vi "32路模拟量输入.vi"() -> ()   [LabVIEW 2010]
uses:
  全局量/全局_配置.vi
panel:
  in  "同步_1":i32
  in  "数组_反馈值":dbl[][](array[numeric])
  in  "第几个数据":i32
  in  "第几组数据":i32
  out "数组_AD幅值":sgl[](array[numeric])
  out "数组_DSP幅值":sgl[](array[numeric])
  in  "数组_设定值":dbl[][](array[numeric])
  in  "数组_选择":bool[](array[boolean])
  out "light_32":bool
  out "light_31":bool
  out "light_30":bool
  out "light_29":bool
  out "light_28":bool
  out "light_27":bool
  out "light_26":bool
  out "light_25":bool
  out "light_24":bool
  out "light_23":bool
  out "light_22":bool
  out "light_21":bool
  out "light_20":bool
  out "light_19":bool
  out "light_18":bool
  out "light_17":bool
  out "Analog_back":string[][](table) caption="表格"
  in  "A_32":bool
  in  "A_31":bool
  in  "A_30":bool
  in  "A_29":bool
  in  "A_28":bool
  in  "A_27":bool
  in  "A_26":bool
  in  "A_25":bool
  in  "A_24":bool
  in  "A_23":bool
  in  "A_22":bool
  in  "A_21":bool
  in  "A_20":bool
  in  "A_19":bool
  in  "A_18":bool
  in  "A_17":bool
  out "合格？":bool[][](array[boolean])
  out "测试结论":string
  out "light_16":bool
  out "light_15":bool
  out "light_14":bool
  out "light_13":bool
  out "light_12":bool
  out "light_11":bool
  out "light_10":bool
  out "light_9":bool
  out "light_8":bool
  out "light_7":bool
  out "light_6":bool
  out "light_5":bool
  out "light_4":bool
  out "light_3":bool
  out "light_2":bool
  out "light_1":bool
  out "退出？":bool
  in  "btn_反选":bool
  in  "btn_全选":bool
  in  "A_16":bool
  in  "A_15":bool
  in  "A_14":bool
  in  "A_13":bool
  in  "A_12":bool
  in  "A_11":bool
  in  "A_10":bool
  in  "A_9":bool
  in  "A_8":bool
  in  "A_7":bool
  in  "A_6":bool
  in  "A_5":bool
  in  "A_4":bool
  in  "A_3":bool
  in  "A_2":bool
  in  "A_1":bool
  in  "btn_取消":bool
  in  "btn_开始测试":bool
  in  "Analog_IN":string[][](table) caption="表格"
  out "Analog_WC":string[][](table) caption="表格"
  # "模拟量选择及输入值（V）"
  # "模拟量反馈值（V）"
  # "模拟量误差值（%）"
  # "测试结论："
  # "从0开始"
  # "从1开始,第0列没有使用"
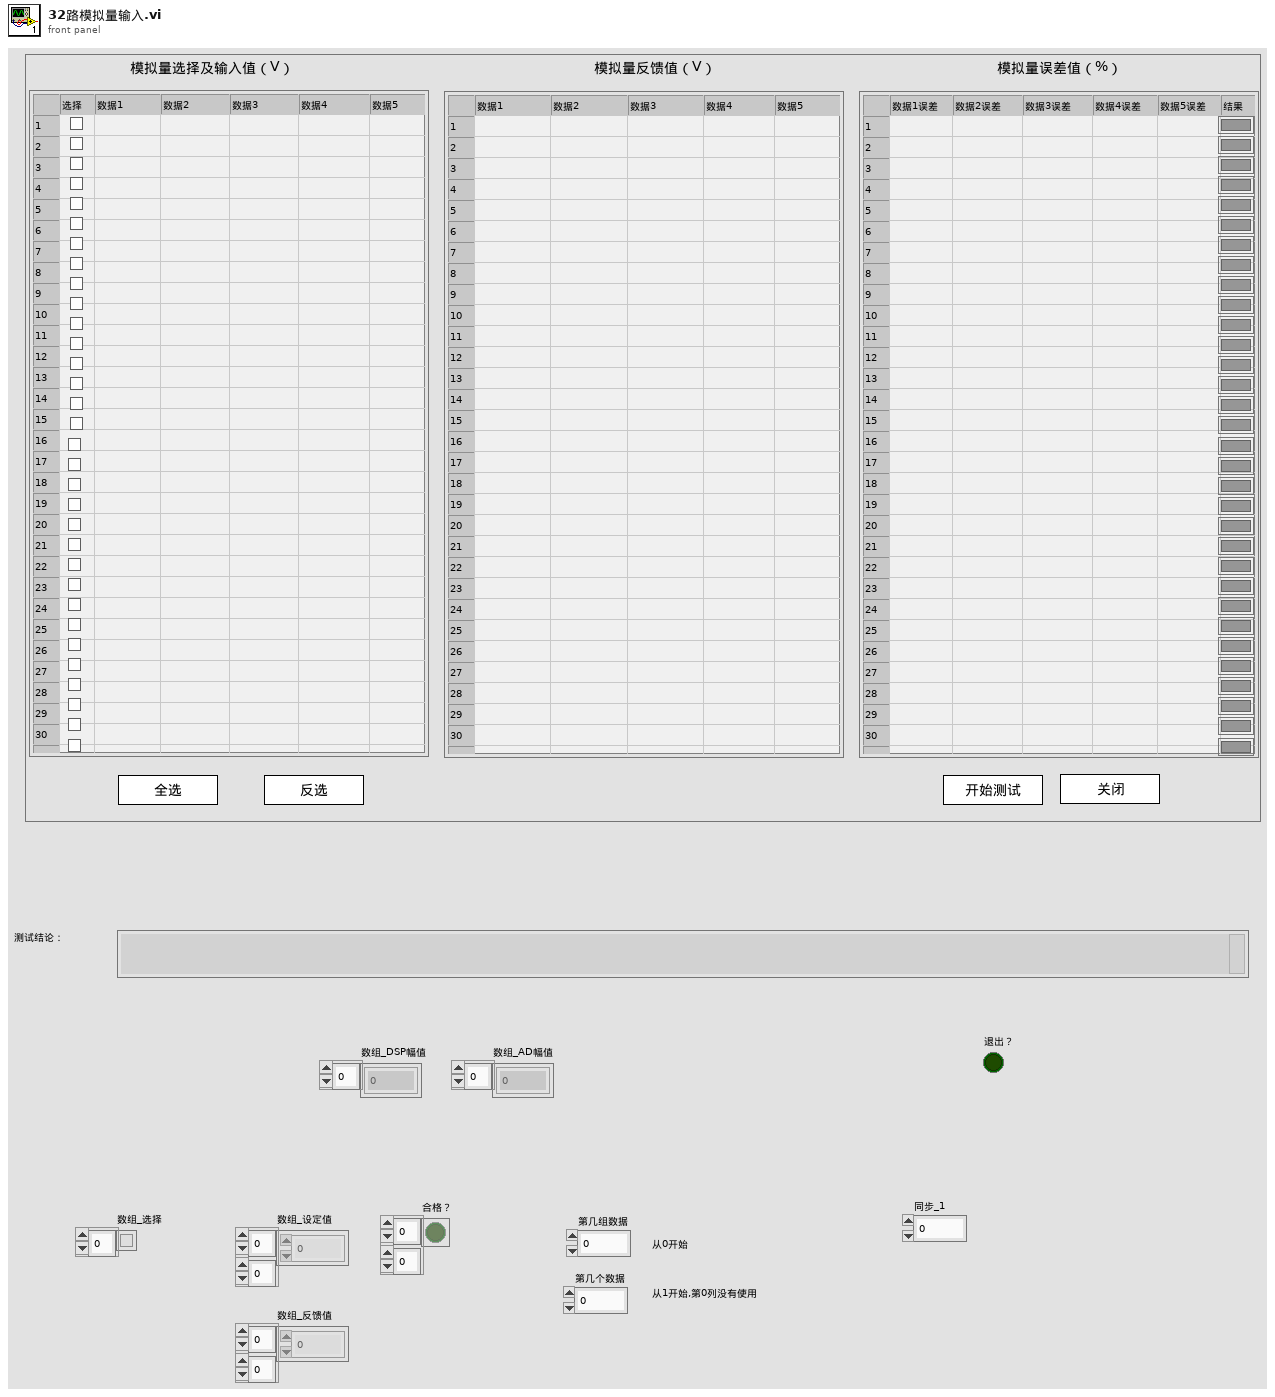
[diagram p1: front panel]
types:
  T1 = enum8{"Enabled", "Disabled", "Disabled and Grayed Out"}
  T2 = cluster{"数字量输入信号路数":u32, "数字量输出信号路数":u32, "DSP模拟量输入信号路数":u32, "DSP模拟量输入信号幅值":u32, "AD模拟量输入信号路数":u32, "AD模拟量输入信号幅值":u32, "RS232端口":i32, "RS232通信路数":u32, "RS232波特率":u32, "RS485端口":u32, "RS485通信路数":u32, "RS485波特率":u32, "CAN通信路数":i32, "CAN波特率":u32, "以太网选择?":bool, "控制板IP":string, "以太网端口":u32}
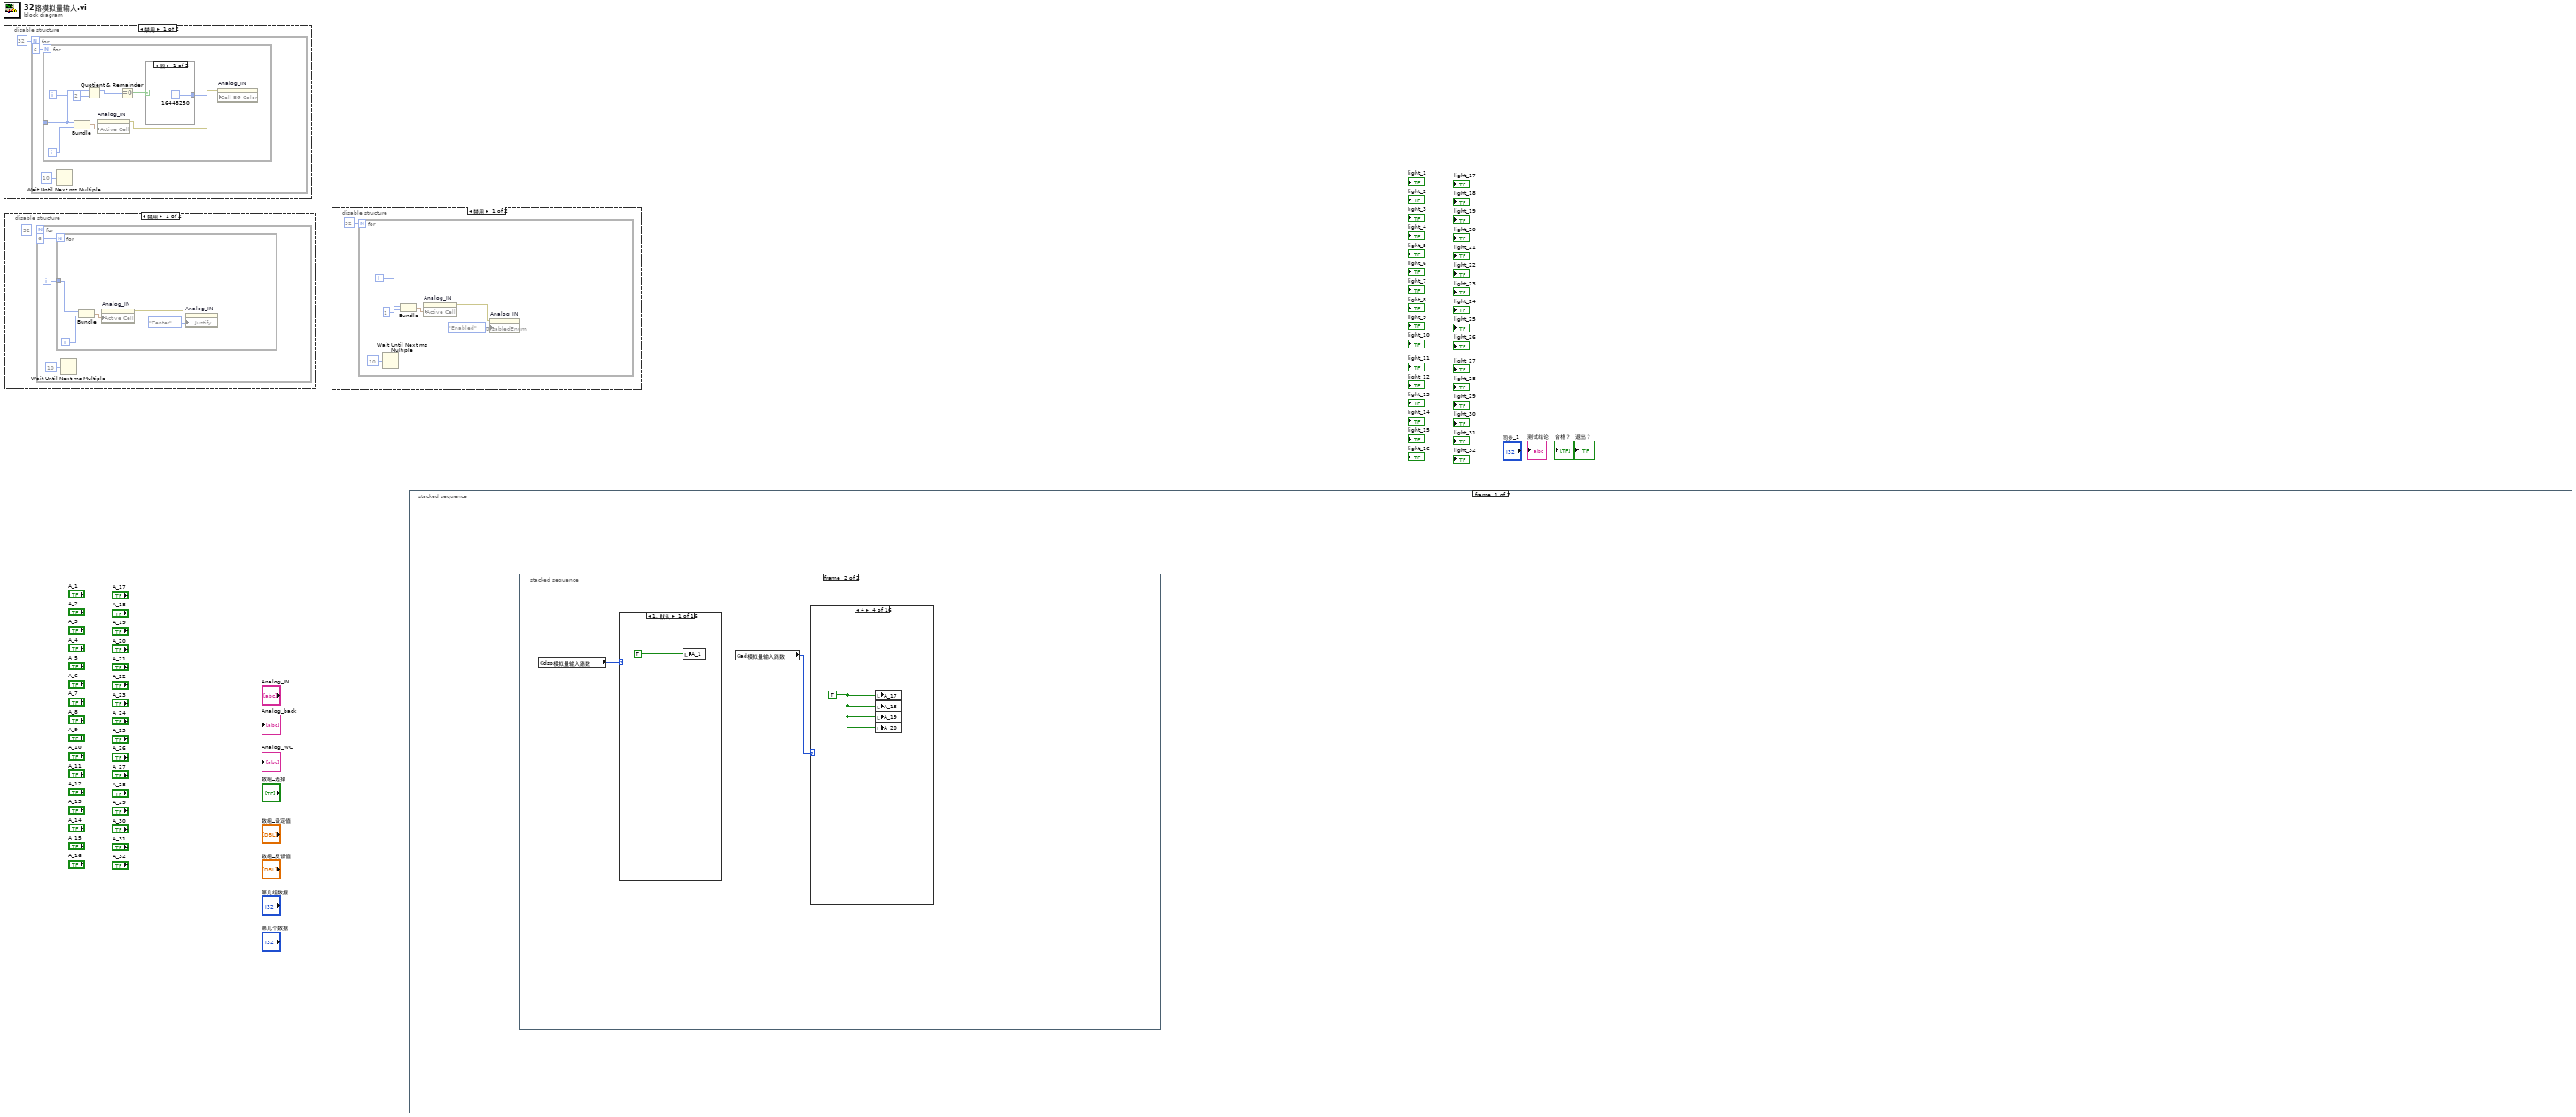
[diagram p0: block diagram]
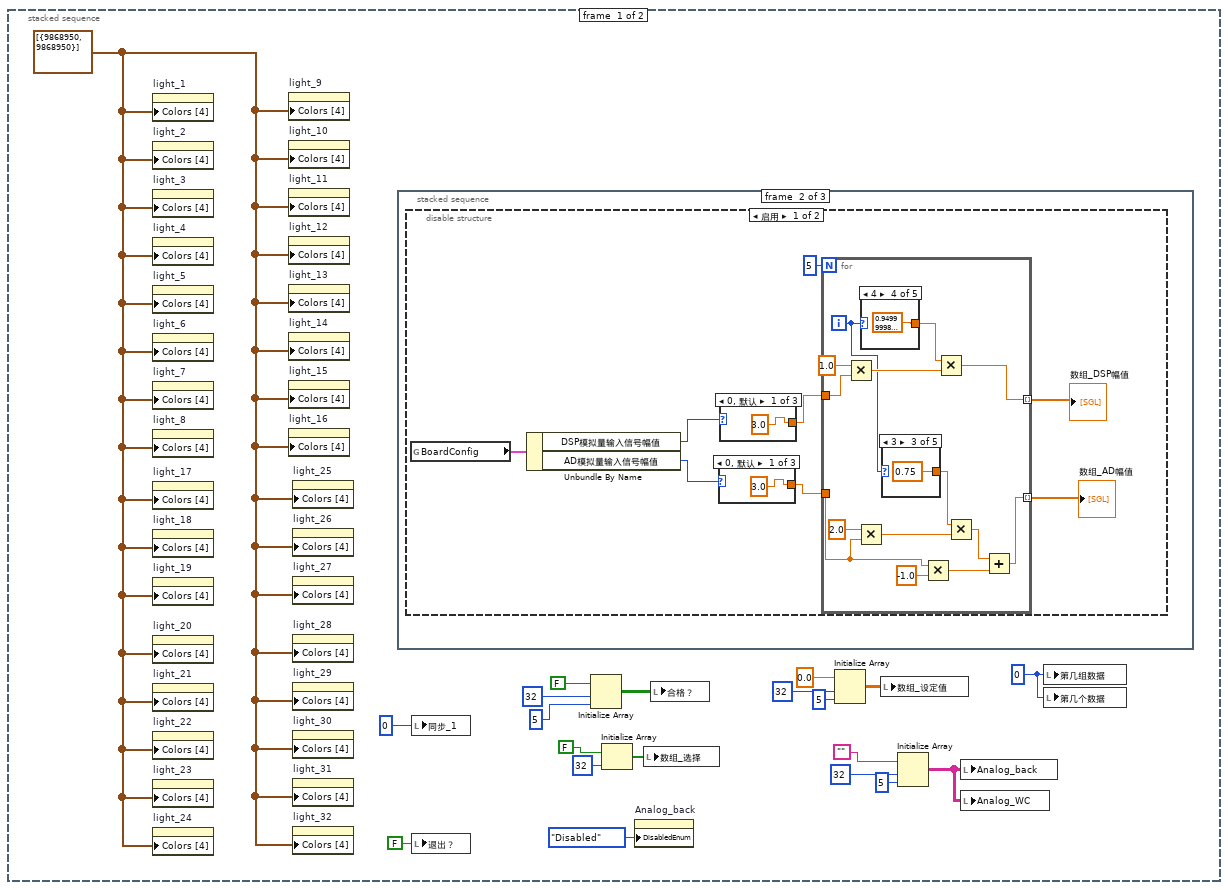
[diagram p2: hidden frame]
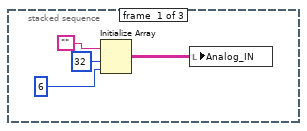
[diagram p3: hidden frame]
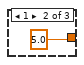
[diagram p4: hidden frame]
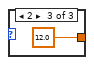
[diagram p5: hidden frame]
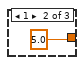
[diagram p6: hidden frame]
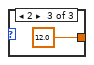
[diagram p7: hidden frame]
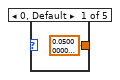
[diagram p8: hidden frame]
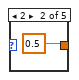
[diagram p9: hidden frame]
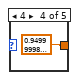
[diagram p10: hidden frame]
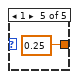
[diagram p11: hidden frame]
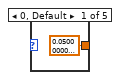
[diagram p12: hidden frame]
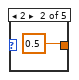
[diagram p13: hidden frame]
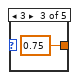
[diagram p14: hidden frame]
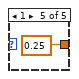
[diagram p15: hidden frame]
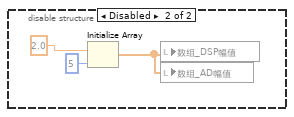
[diagram p16: hidden frame]
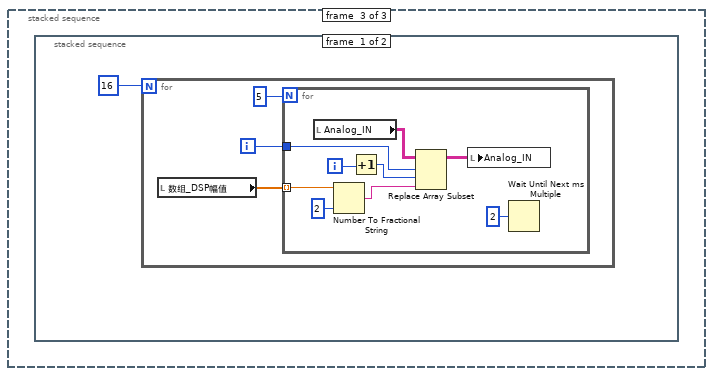
[diagram p17: hidden frame]
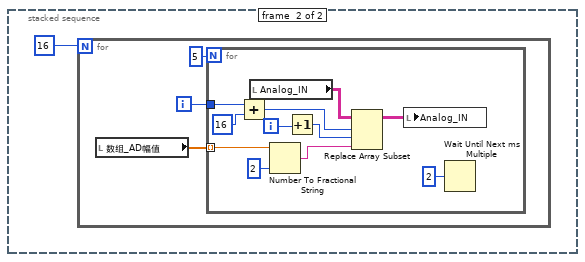
[diagram p18: hidden frame]
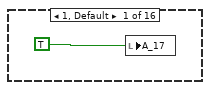
[diagram p19: hidden frame]
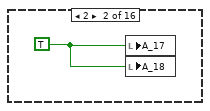
[diagram p20: hidden frame]
diagram:
  n1 = disable-structure shown="禁用" {
    frame Disabled {
      n2 = for {
        N: 32 -> [_]
        i -> [w3]
        n3 = for {
          N: 6 -> [_]
          tunnel: w3 -> [w11]
          i -> [w5]
          n4 = Bundle(w11, w5) -> (w8:cluster{i32, i32})  [unwired: 1 in]
          n5 = Quotient & Remainder(x=w11, y=2) -> (x-y*floor(x/y)=w9:i32)  [unwired: 1 out]
          n6 = property on="Analog_IN" class="Tbl (严格)"("Active Cell"=w8) -> (error out=w7:errorcluster)  [unwired: 2 in, 1 out]
          n7 = Equal To 0?(x=w9) -> (x = 0?=w12:bool)
          n8 = case shown="假" w12 {
            tunnel: [u32 16448250 u32 15723488] -> w6
            frame False {
            }
            frame True {
            }
          }
          n9 = property on="Analog_IN" class="Tbl (严格)"(error in=w7, "Cell BG Color"=w6) -> ()  [unwired: 1 in, 2 out]
        }
        n10 = Wait Until Next ms Multiple(millisecond multiple=u32 10 ("毫秒倍数")) -> ()  [unwired: 1 out]
      }
    }
    frame Enabled {
    }
  }
  n11 = disable-structure shown="禁用" {
    frame Disabled {
      n12 = for {
        N: 32 -> [_]
        i -> [w16]
        n13 = for {
          N: 6 -> [_]
          tunnel: w16 -> [w19]
          i -> [w20]
          n14 = Bundle(w19, w20) -> (w23:cluster{i32, i32})  [unwired: 1 in]
          n15 = property on="Analog_IN" class="Tbl (严格)"("Active Cell"=w23) -> (error out=w21:errorcluster)  [unwired: 2 in, 1 out]
          n16 = property on="Analog_IN" class="Tbl (严格)"(error in=w21, "Justify"=enum16{"Left", "Center", "Right"}."Center" ("活动单元格:单元格对齐")) -> ()  [unwired: 1 in, 2 out]
        }
        n17 = Wait Until Next ms Multiple(millisecond multiple=u32 10 ("毫秒倍数")) -> ()  [unwired: 1 out]
      }
    }
    frame Enabled {
    }
  }
  n18 = disable-structure shown="禁用" {
    frame Disabled {
      n19 = for {
        N: 32 -> [_]
        i -> [w29]
        n20 = Wait Until Next ms Multiple(millisecond multiple=u32 10 ("毫秒倍数")) -> ()  [unwired: 1 out]
        n21 = Bundle(w29, 1) -> (w28:cluster{i32, i32})  [unwired: 1 in]
        n22 = property on="Analog_IN" class="Tbl (严格)"("Active Cell"=w28) -> (error out=w25:errorcluster)  [unwired: 2 in, 1 out]
        n23 = property on="Analog_IN" class="Tbl (严格)"(error in=w25, "DisabledEnum"=T1."Enabled" ("禁用")) -> ()  [unwired: 1 in, 2 out]
      }
    }
    frame Enabled {
    }
  }
  n24 = stacked-sequence {
    frame #0 {
      n25 = stacked-sequence {
        frame #0 {
          w31 = 0 ("第几组数据")
          w46 = cluster{u32, u32}[] [{9868950, 9868950}]
          n26 = property on="light_1" class="Bool (严格)"("Colors [4]"=w46) -> ()  [unwired: 2 in, 2 out]
          n27 = property on="light_2" class="Bool (严格)"("Colors [4]"=w46) -> ()  [unwired: 2 in, 2 out]
          n28 = property on="light_3" class="Bool (严格)"("Colors [4]"=w46) -> ()  [unwired: 2 in, 2 out]
          n29 = property on="light_4" class="Bool (严格)"("Colors [4]"=w46) -> ()  [unwired: 2 in, 2 out]
          n30 = property on="light_5" class="Bool (严格)"("Colors [4]"=w46) -> ()  [unwired: 2 in, 2 out]
          n31 = property on="light_6" class="Bool (严格)"("Colors [4]"=w46) -> ()  [unwired: 2 in, 2 out]
          n32 = property on="light_7" class="Bool (严格)"("Colors [4]"=w46) -> ()  [unwired: 2 in, 2 out]
          n33 = property on="light_8" class="Bool (严格)"("Colors [4]"=w46) -> ()  [unwired: 2 in, 2 out]
          n34 = property on="light_17" class="Bool (严格)"("Colors [4]"=w46) -> ()  [unwired: 2 in, 2 out]
          n35 = property on="light_18" class="Bool (严格)"("Colors [4]"=w46) -> ()  [unwired: 2 in, 2 out]
          n36 = property on="light_19" class="Bool (严格)"("Colors [4]"=w46) -> ()  [unwired: 2 in, 2 out]
          n37 = property on="light_20" class="Bool (严格)"("Colors [4]"=w46) -> ()  [unwired: 2 in, 2 out]
          n38 = property on="light_21" class="Bool (严格)"("Colors [4]"=w46) -> ()  [unwired: 2 in, 2 out]
          n39 = property on="light_22" class="Bool (严格)"("Colors [4]"=w46) -> ()  [unwired: 2 in, 2 out]
          n40 = property on="light_23" class="Bool (严格)"("Colors [4]"=w46) -> ()  [unwired: 2 in, 2 out]
          n41 = property on="light_24" class="Bool (严格)"("Colors [4]"=w46) -> ()  [unwired: 2 in, 2 out]
          n42 = property on="light_9" class="Bool (严格)"("Colors [4]"=w46) -> ()  [unwired: 2 in, 2 out]
          n43 = property on="light_10" class="Bool (严格)"("Colors [4]"=w46) -> ()  [unwired: 2 in, 2 out]
          n44 = property on="light_11" class="Bool (严格)"("Colors [4]"=w46) -> ()  [unwired: 2 in, 2 out]
          n45 = property on="light_12" class="Bool (严格)"("Colors [4]"=w46) -> ()  [unwired: 2 in, 2 out]
          n46 = property on="light_13" class="Bool (严格)"("Colors [4]"=w46) -> ()  [unwired: 2 in, 2 out]
          n47 = property on="light_14" class="Bool (严格)"("Colors [4]"=w46) -> ()  [unwired: 2 in, 2 out]
          n48 = property on="light_15" class="Bool (严格)"("Colors [4]"=w46) -> ()  [unwired: 2 in, 2 out]
          n49 = property on="light_16" class="Bool (严格)"("Colors [4]"=w46) -> ()  [unwired: 2 in, 2 out]
          n50 = property on="light_25" class="Bool (严格)"("Colors [4]"=w46) -> ()  [unwired: 2 in, 2 out]
          n51 = property on="light_26" class="Bool (严格)"("Colors [4]"=w46) -> ()  [unwired: 2 in, 2 out]
          n52 = property on="light_27" class="Bool (严格)"("Colors [4]"=w46) -> ()  [unwired: 2 in, 2 out]
          n53 = property on="light_28" class="Bool (严格)"("Colors [4]"=w46) -> ()  [unwired: 2 in, 2 out]
          n54 = property on="light_29" class="Bool (严格)"("Colors [4]"=w46) -> ()  [unwired: 2 in, 2 out]
          n55 = property on="light_30" class="Bool (严格)"("Colors [4]"=w46) -> ()  [unwired: 2 in, 2 out]
          n56 = property on="light_31" class="Bool (严格)"("Colors [4]"=w46) -> ()  [unwired: 2 in, 2 out]
          n57 = property on="light_32" class="Bool (严格)"("Colors [4]"=w46) -> ()  [unwired: 2 in, 2 out]
          n58 = stacked-sequence {
            frame #0 {
              n59 = Initialize Array("", 32 ("维数大小"), 6 ("维数大小")) -> (w51:string[][])
              n60 = local write "Analog_IN"(w51) -> ()
            }
            frame #1 {
              n61 = disable-structure shown="启用" {
                frame Enabled {
                  n62 = global read "全局_配置.vi" "BoardConfig"() -> (w59:T2)
                  n63 = Unbundle By Name(w59) -> ("DSP模拟量输入信号幅值"=w58:u32, "AD模拟量输入信号幅值"=w57:u32)
                  n64 = case shown="0, 默认" w57 {
                    tunnel: [sgl 3.0 sgl 5.0 sgl 12.0] -> w55
                    frame 0, Default {
                    }
                    frame 1 {
                    }
                    frame 2 {
                    }
                  }
                  n65 = case shown="0, 默认" w58 {
                    tunnel: [sgl 3.0 sgl 5.0 sgl 12.0] -> w56
                    frame 0, Default {
                    }
                    frame 1 {
                    }
                    frame 2 {
                    }
                  }
                  n66 = for {
                    N: 5 -> [_]
                    tunnel: w56 -> [w82]
                    tunnel: w55 -> [w74]
                    tunnel: [w69] -> w61 mode=indexing
                    tunnel: [w72] -> w60 mode=indexing
                    i -> [w71]
                    n67 = Multiply(x=sgl 1.0, y=w82) -> (x*y=w80:sgl)
                    n68 = Multiply(x=sgl 2.0, y=w74) -> (x*y=w78:sgl)
                    n69 = case shown="4" w71 {
                      tunnel: [sgl 0.05 sgl 0.5 sgl 0.75 sgl 0.95 sgl 0.25] -> w73
                      frame 0, Default {
                      }
                      frame 2 {
                      }
                      frame 3 {
                      }
                      frame 4 {
                      }
                      frame 1 {
                      }
                    }
                    n70 = case shown="3" w71 {
                      tunnel: [sgl 0.05 sgl 0.5 sgl 0.75 sgl 0.95 sgl 0.25] -> w70
                      frame 0, Default {
                      }
                      frame 2 {
                      }
                      frame 3 {
                      }
                      frame 4 {
                      }
                      frame 1 {
                      }
                    }
                    n71 = Multiply(x=w74, y=sgl -1.0) -> (x*y=w76:sgl)
                    n72 = Multiply(x=w73, y=w80) -> (x*y=w69:sgl)
                    n73 = Multiply(x=w70, y=w78) -> (x*y=w79:sgl)
                    n74 = Add(x=w79, y=w76) -> (x+y=w72:sgl)
                  }
                  "数组_DSP幅值" <- w61
                  "数组_AD幅值" <- w60
                }
                frame Disabled {
                  n75 = Initialize Array(sgl 2.0, 5 ("维数大小")) -> (w95:sgl[])
                  n76 = local write "数组_DSP幅值"(w95) -> ()
                  n77 = local write "数组_AD幅值"(w95) -> ()
                }
              }
            }
            frame #2 {
              n78 = stacked-sequence {
                frame #0 {
                  n79 = for {
                    N: 16 -> [_]
                    i -> [w97]
                    n80 = local read "数组_DSP幅值"() -> (w98:sgl[])
                    n81 = for {
                      N: 5 -> [_]
                      tunnel: w98 -> [w105] mode=indexing
                      tunnel: w97 -> [w104]
                      i -> [w102]
                      n82 = local read "Analog_IN"() -> (w108:string[][])
                      n83 = Number To Fractional String(number=w105, precision (6)=i16 2 ("精度(6)")) -> (F-format string=w103:string)  [unwired: 2 in]
                      n84 = Increment(x=w102) -> (x+1=w101:i32)
                      n85 = Replace Array Subset(array=w108, new element=w103, index (row)=w104, index (col)=w101) -> (w107:string[][])
                      n86 = local write "Analog_IN"(w107) -> ()
                      n87 = Wait Until Next ms Multiple(millisecond multiple=u32 2 ("毫秒倍数")) -> ()  [unwired: 1 out]
                    }
                  }
                }
                frame #1 {
                  n88 = for {
                    N: 16 -> [_]
                    i -> [w111]
                    n89 = local read "数组_AD幅值"() -> (w110:sgl[])
                    n90 = for {
                      N: 5 -> [_]
                      tunnel: w110 -> [w120] mode=indexing
                      tunnel: w111 -> [w115]
                      i -> [w118]
                      n91 = Add(x=w115, y=16) -> (x+y=w113:i32)
                      n92 = local read "Analog_IN"() -> (w123:string[][])
                      n93 = Number To Fractional String(number=w120, precision (6)=i16 2 ("精度(6)")) -> (F-format string=w119:string)  [unwired: 2 in]
                      n94 = Increment(x=w118) -> (x+1=w117:i32)
                      n95 = Replace Array Subset(array=w123, new element=w119, index (row)=w113, index (col)=w117) -> (w122:string[][])
                      n96 = local write "Analog_IN"(w122) -> ()
                      n97 = Wait Until Next ms Multiple(millisecond multiple=u32 2 ("毫秒倍数")) -> ()  [unwired: 1 out]
                    }
                  }
                }
              }
            }
          }
          n98 = local write "同步_1"(0 ("同步_2")) -> ()
          n99 = local write "退出？"(FALSE ("退出？")) -> ()
          n100 = Initialize Array(FALSE, 32 ("维数大小"), 5 ("维数大小")) -> (w47:bool[][])
          n101 = Initialize Array(FALSE, 32 ("维数大小")) -> (w35:bool[])
          n102 = property on="Analog_back" class="Tbl (严格)"("DisabledEnum"=T1."Disabled" ("禁用")) -> ()  [unwired: 2 in, 2 out]
          n103 = local write "数组_选择"(w35) -> ()
          n104 = local write "合格？"(w47) -> ()
          n105 = Initialize Array(0.0, 32 ("维数大小"), 5 ("维数大小")) -> (w38:dbl[][])
          n106 = local write "数组_设定值"(w38) -> ()
          n107 = Initialize Array("", 32 ("维数大小"), 5 ("维数大小")) -> (w42:string[][])
          n108 = local write "Analog_back"(w42) -> ()
          n109 = local write "Analog_WC"(w42) -> ()
          n110 = local write "第几组数据"(w31) -> ()
          n111 = local write "第几个数据"(w31) -> ()
        }
        frame #1 {
          n112 = global read "全局_配置.vi" "dsp模拟量输入路数"() -> (w125:u32)
          n113 = case shown="1, 默认" w125 {
            frame 1, Default {
              n114 = local write "A_1"(TRUE ("单选_AD_1")) -> ()
            }
            frame 2 {
              w143 = TRUE ("单选_AD_1")
              n115 = local write "A_1"(w143) -> ()
              n116 = local write "A_2"(w143) -> ()
            }
            frame 3 {
              w144 = TRUE ("单选_AD_1")
              n117 = local write "A_1"(w144) -> ()
              n118 = local write "A_2"(w144) -> ()
              n119 = local write "A_3"(w144) -> ()
            }
            frame 4 {
              w145 = TRUE ("单选_AD_1")
              n120 = local write "A_1"(w145) -> ()
              n121 = local write "A_2"(w145) -> ()
              n122 = local write "A_3"(w145) -> ()
              n123 = local write "A_4"(w145) -> ()
            }
            frame 5 {
              w146 = TRUE ("单选_AD_1")
              n124 = local write "A_1"(w146) -> ()
              n125 = local write "A_2"(w146) -> ()
              n126 = local write "A_3"(w146) -> ()
              n127 = local write "A_4"(w146) -> ()
              n128 = local write "A_5"(w146) -> ()
            }
            frame 6 {
              w147 = TRUE ("单选_AD_1")
              n129 = local write "A_1"(w147) -> ()
              n130 = local write "A_2"(w147) -> ()
              n131 = local write "A_3"(w147) -> ()
              n132 = local write "A_4"(w147) -> ()
              n133 = local write "A_5"(w147) -> ()
              n134 = local write "A_6"(w147) -> ()
            }
            frame 7 {
              w148 = TRUE ("单选_AD_1")
              n135 = local write "A_1"(w148) -> ()
              n136 = local write "A_2"(w148) -> ()
              n137 = local write "A_3"(w148) -> ()
              n138 = local write "A_4"(w148) -> ()
              n139 = local write "A_5"(w148) -> ()
              n140 = local write "A_6"(w148) -> ()
              n141 = local write "A_7"(w148) -> ()
            }
            frame 8 {
              w149 = TRUE ("单选_AD_1")
              n142 = local write "A_1"(w149) -> ()
              n143 = local write "A_2"(w149) -> ()
              n144 = local write "A_3"(w149) -> ()
              n145 = local write "A_4"(w149) -> ()
              n146 = local write "A_5"(w149) -> ()
              n147 = local write "A_6"(w149) -> ()
              n148 = local write "A_7"(w149) -> ()
              n149 = local write "A_8"(w149) -> ()
            }
            frame 9 {
              w150 = TRUE ("单选_AD_1")
              n150 = local write "A_1"(w150) -> ()
              n151 = local write "A_2"(w150) -> ()
              n152 = local write "A_3"(w150) -> ()
              n153 = local write "A_4"(w150) -> ()
              n154 = local write "A_5"(w150) -> ()
              n155 = local write "A_6"(w150) -> ()
              n156 = local write "A_7"(w150) -> ()
              n157 = local write "A_8"(w150) -> ()
              n158 = local write "A_9"(w150) -> ()
            }
            frame 10 {
              w151 = TRUE ("单选_AD_1")
              n159 = local write "A_1"(w151) -> ()
              n160 = local write "A_2"(w151) -> ()
              n161 = local write "A_3"(w151) -> ()
              n162 = local write "A_4"(w151) -> ()
              n163 = local write "A_5"(w151) -> ()
              n164 = local write "A_6"(w151) -> ()
              n165 = local write "A_7"(w151) -> ()
              n166 = local write "A_8"(w151) -> ()
              n167 = local write "A_9"(w151) -> ()
              n168 = local write "A_10"(w151) -> ()
            }
            frame 11 {
              w152 = TRUE ("单选_AD_1")
              n169 = local write "A_1"(w152) -> ()
              n170 = local write "A_2"(w152) -> ()
              n171 = local write "A_3"(w152) -> ()
              n172 = local write "A_4"(w152) -> ()
              n173 = local write "A_5"(w152) -> ()
              n174 = local write "A_6"(w152) -> ()
              n175 = local write "A_7"(w152) -> ()
              n176 = local write "A_8"(w152) -> ()
              n177 = local write "A_9"(w152) -> ()
              n178 = local write "A_10"(w152) -> ()
              n179 = local write "A_11"(w152) -> ()
            }
            frame 12 {
              w153 = TRUE ("单选_AD_1")
              n180 = local write "A_1"(w153) -> ()
              n181 = local write "A_2"(w153) -> ()
              n182 = local write "A_3"(w153) -> ()
              n183 = local write "A_4"(w153) -> ()
              n184 = local write "A_5"(w153) -> ()
              n185 = local write "A_6"(w153) -> ()
              n186 = local write "A_7"(w153) -> ()
              n187 = local write "A_8"(w153) -> ()
              n188 = local write "A_9"(w153) -> ()
              n189 = local write "A_10"(w153) -> ()
              n190 = local write "A_11"(w153) -> ()
              n191 = local write "A_12"(w153) -> ()
            }
            frame 13 {
              w154 = TRUE ("单选_AD_1")
              n192 = local write "A_1"(w154) -> ()
              n193 = local write "A_2"(w154) -> ()
              n194 = local write "A_3"(w154) -> ()
              n195 = local write "A_4"(w154) -> ()
              n196 = local write "A_5"(w154) -> ()
              n197 = local write "A_6"(w154) -> ()
              n198 = local write "A_7"(w154) -> ()
              n199 = local write "A_8"(w154) -> ()
              n200 = local write "A_9"(w154) -> ()
              n201 = local write "A_10"(w154) -> ()
              n202 = local write "A_11"(w154) -> ()
              n203 = local write "A_12"(w154) -> ()
              n204 = local write "A_13"(w154) -> ()
            }
            frame 14 {
              w155 = TRUE ("单选_AD_1")
              n205 = local write "A_1"(w155) -> ()
              n206 = local write "A_2"(w155) -> ()
              n207 = local write "A_3"(w155) -> ()
              n208 = local write "A_4"(w155) -> ()
              n209 = local write "A_5"(w155) -> ()
              n210 = local write "A_6"(w155) -> ()
              n211 = local write "A_7"(w155) -> ()
              n212 = local write "A_8"(w155) -> ()
              n213 = local write "A_9"(w155) -> ()
              n214 = local write "A_10"(w155) -> ()
              n215 = local write "A_11"(w155) -> ()
              n216 = local write "A_12"(w155) -> ()
              n217 = local write "A_13"(w155) -> ()
              n218 = local write "A_14"(w155) -> ()
            }
            frame 15 {
              w156 = TRUE ("单选_AD_1")
              n219 = local write "A_1"(w156) -> ()
              n220 = local write "A_2"(w156) -> ()
              n221 = local write "A_3"(w156) -> ()
              n222 = local write "A_4"(w156) -> ()
              n223 = local write "A_5"(w156) -> ()
              n224 = local write "A_6"(w156) -> ()
              n225 = local write "A_7"(w156) -> ()
              n226 = local write "A_8"(w156) -> ()
              n227 = local write "A_9"(w156) -> ()
              n228 = local write "A_10"(w156) -> ()
              n229 = local write "A_11"(w156) -> ()
              n230 = local write "A_12"(w156) -> ()
              n231 = local write "A_13"(w156) -> ()
              n232 = local write "A_14"(w156) -> ()
              n233 = local write "A_15"(w156) -> ()
            }
            frame 16 {
              w157 = TRUE ("单选_AD_1")
              n234 = local write "A_1"(w157) -> ()
              n235 = local write "A_2"(w157) -> ()
              n236 = local write "A_3"(w157) -> ()
              n237 = local write "A_4"(w157) -> ()
              n238 = local write "A_5"(w157) -> ()
              n239 = local write "A_6"(w157) -> ()
              n240 = local write "A_7"(w157) -> ()
              n241 = local write "A_8"(w157) -> ()
              n242 = local write "A_9"(w157) -> ()
              n243 = local write "A_10"(w157) -> ()
              n244 = local write "A_11"(w157) -> ()
              n245 = local write "A_12"(w157) -> ()
              n246 = local write "A_13"(w157) -> ()
              n247 = local write "A_14"(w157) -> ()
              n248 = local write "A_15"(w157) -> ()
              n249 = local write "A_16"(w157) -> ()
            }
          }
          n250 = global read "全局_配置.vi" "ad模拟量输入路数"() -> (w124:u32)
          n251 = case shown="4" w124 {
            frame 1, Default {
              n252 = local write "A_17"(TRUE ("单选_AD_1")) -> ()
            }
            frame 2 {
              w127 = TRUE ("单选_AD_1")
              n253 = local write "A_17"(w127) -> ()
              n254 = local write "A_18"(w127) -> ()
            }
            frame 3 {
              w128 = TRUE ("单选_AD_1")
              n255 = local write "A_17"(w128) -> ()
              n256 = local write "A_18"(w128) -> ()
              n257 = local write "A_19"(w128) -> ()
            }
            frame 4 {
              w129 = TRUE ("单选_AD_1")
              n258 = local write "A_17"(w129) -> ()
              n259 = local write "A_18"(w129) -> ()
              n260 = local write "A_19"(w129) -> ()
              n261 = local write "A_20"(w129) -> ()
            }
            frame 5 {
              w130 = TRUE ("单选_AD_1")
              n262 = local write "A_17"(w130) -> ()
              n263 = local write "A_18"(w130) -> ()
              n264 = local write "A_19"(w130) -> ()
              n265 = local write "A_20"(w130) -> ()
              n266 = local write "A_21"(w130) -> ()
            }
            frame 6 {
              w131 = TRUE ("单选_AD_1")
              n267 = local write "A_17"(w131) -> ()
              n268 = local write "A_18"(w131) -> ()
              n269 = local write "A_19"(w131) -> ()
              n270 = local write "A_20"(w131) -> ()
              n271 = local write "A_21"(w131) -> ()
              n272 = local write "A_22"(w131) -> ()
            }
            frame 7 {
              w132 = TRUE ("单选_AD_1")
              n273 = local write "A_17"(w132) -> ()
              n274 = local write "A_18"(w132) -> ()
              n275 = local write "A_19"(w132) -> ()
              n276 = local write "A_20"(w132) -> ()
              n277 = local write "A_21"(w132) -> ()
              n278 = local write "A_22"(w132) -> ()
              n279 = local write "A_23"(w132) -> ()
            }
            frame 8 {
              w133 = TRUE ("单选_AD_1")
              n280 = local write "A_17"(w133) -> ()
              n281 = local write "A_18"(w133) -> ()
              n282 = local write "A_19"(w133) -> ()
              n283 = local write "A_20"(w133) -> ()
              n284 = local write "A_21"(w133) -> ()
              n285 = local write "A_22"(w133) -> ()
              n286 = local write "A_23"(w133) -> ()
              n287 = local write "A_24"(w133) -> ()
            }
            frame 9 {
              w134 = TRUE ("单选_AD_1")
              n288 = local write "A_17"(w134) -> ()
              n289 = local write "A_18"(w134) -> ()
              n290 = local write "A_19"(w134) -> ()
              n291 = local write "A_20"(w134) -> ()
              n292 = local write "A_21"(w134) -> ()
              n293 = local write "A_22"(w134) -> ()
              n294 = local write "A_23"(w134) -> ()
              n295 = local write "A_24"(w134) -> ()
              n296 = local write "A_25"(w134) -> ()
            }
            frame 10 {
              w135 = TRUE ("单选_AD_1")
              n297 = local write "A_17"(w135) -> ()
              n298 = local write "A_18"(w135) -> ()
              n299 = local write "A_19"(w135) -> ()
              n300 = local write "A_20"(w135) -> ()
              n301 = local write "A_21"(w135) -> ()
              n302 = local write "A_22"(w135) -> ()
              n303 = local write "A_23"(w135) -> ()
              n304 = local write "A_24"(w135) -> ()
              n305 = local write "A_25"(w135) -> ()
              n306 = local write "A_26"(w135) -> ()
            }
            frame 11 {
              w136 = TRUE ("单选_AD_1")
              n307 = local write "A_17"(w136) -> ()
              n308 = local write "A_18"(w136) -> ()
              n309 = local write "A_19"(w136) -> ()
              n310 = local write "A_20"(w136) -> ()
              n311 = local write "A_21"(w136) -> ()
              n312 = local write "A_22"(w136) -> ()
              n313 = local write "A_23"(w136) -> ()
              n314 = local write "A_24"(w136) -> ()
              n315 = local write "A_25"(w136) -> ()
              n316 = local write "A_26"(w136) -> ()
              n317 = local write "A_27"(w136) -> ()
            }
            frame 12 {
              w137 = TRUE ("单选_AD_1")
              n318 = local write "A_17"(w137) -> ()
              n319 = local write "A_18"(w137) -> ()
              n320 = local write "A_19"(w137) -> ()
              n321 = local write "A_20"(w137) -> ()
              n322 = local write "A_21"(w137) -> ()
              n323 = local write "A_22"(w137) -> ()
              n324 = local write "A_23"(w137) -> ()
              n325 = local write "A_24"(w137) -> ()
              n326 = local write "A_25"(w137) -> ()
              n327 = local write "A_26"(w137) -> ()
              n328 = local write "A_27"(w137) -> ()
              n329 = local write "A_28"(w137) -> ()
            }
            frame 13 {
              w138 = TRUE ("单选_AD_1")
              n330 = local write "A_17"(w138) -> ()
              n331 = local write "A_18"(w138) -> ()
              n332 = local write "A_19"(w138) -> ()
              n333 = local write "A_20"(w138) -> ()
              n334 = local write "A_21"(w138) -> ()
              n335 = local write "A_22"(w138) -> ()
              n336 = local write "A_23"(w138) -> ()
              n337 = local write "A_24"(w138) -> ()
              n338 = local write "A_25"(w138) -> ()
              n339 = local write "A_26"(w138) -> ()
              n340 = local write "A_27"(w138) -> ()
              n341 = local write "A_28"(w138) -> ()
              n342 = local write "A_29"(w138) -> ()
            }
            frame 14 {
              w139 = TRUE ("单选_AD_1")
              n343 = local write "A_17"(w139) -> ()
              n344 = local write "A_18"(w139) -> ()
              n345 = local write "A_19"(w139) -> ()
              n346 = local write "A_20"(w139) -> ()
              n347 = local write "A_21"(w139) -> ()
              n348 = local write "A_22"(w139) -> ()
              n349 = local write "A_23"(w139) -> ()
              n350 = local write "A_24"(w139) -> ()
              n351 = local write "A_25"(w139) -> ()
              n352 = local write "A_26"(w139) -> ()
              n353 = local write "A_27"(w139) -> ()
              n354 = local write "A_28"(w139) -> ()
              n355 = local write "A_29"(w139) -> ()
              n356 = local write "A_30"(w139) -> ()
            }
            frame 15 {
              w140 = TRUE ("单选_AD_1")
              n357 = local write "A_17"(w140) -> ()
              n358 = local write "A_18"(w140) -> ()
              n359 = local write "A_19"(w140) -> ()
              n360 = local write "A_20"(w140) -> ()
              n361 = local write "A_21"(w140) -> ()
              n362 = local write "A_22"(w140) -> ()
              n363 = local write "A_23"(w140) -> ()
              n364 = local write "A_24"(w140) -> ()
              n365 = local write "A_25"(w140) -> ()
              n366 = local write "A_26"(w140) -> ()
              n367 = local write "A_27"(w140) -> ()
              n368 = local write "A_28"(w140) -> ()
              n369 = local write "A_29"(w140) -> ()
              n370 = local write "A_30"(w140) -> ()
              n371 = local write "A_31"(w140) -> ()
            }
            frame 16 {
              w141 = TRUE ("单选_AD_1")
              n372 = local write "A_17"(w141) -> ()
              n373 = local write "A_18"(w141) -> ()
              n374 = local write "A_19"(w141) -> ()
              n375 = local write "A_20"(w141) -> ()
              n376 = local write "A_21"(w141) -> ()
              n377 = local write "A_22"(w141) -> ()
              n378 = local write "A_23"(w141) -> ()
              n379 = local write "A_24"(w141) -> ()
              n380 = local write "A_25"(w141) -> ()
              n381 = local write "A_26"(w141) -> ()
              n382 = local write "A_27"(w141) -> ()
              n383 = local write "A_28"(w141) -> ()
              n384 = local write "A_29"(w141) -> ()
              n385 = local write "A_30"(w141) -> ()
              n386 = local write "A_31"(w141) -> ()
              n387 = local write "A_32"(w141) -> ()
            }
          }
        }
      }
    }
    frame #1 {
      w159 = "ANumCheck" ("名称（未命名）")
      w161 = "DSPStart" ("名称（未命名）")
      w166 = "ANumCheck" ("名称（未命名）")
      w169 = "DSPStart" ("名称（未命名）")
      n388 = Obtain Notifier(name (unnamed)=w161, notification data type=w161) -> (notifier out=w160:refnum<notifier>)  [unwired: 2 in, 2 out]
      n389 = while {
        tunnel: w160 -> [w435]
        stop <- w436 stop-if-true
        n390 = event shown="[4] \"btn_全选\": 值改变" {
          selector: _ -> [_ _ _ _ _ _]
          dyn-events: _ -> [_ _ _ _ _ _]
          timeout: _ -> [_ _ _ _ _ _]
          tunnel: [_ TRUE TRUE _ _ _] -> w436
          tunnel: w435 -> [_ _ _ w439 _ _]
          event Timeout {
            n391 = event-data() -> ()  [unwired: 1 in, 2 out]
          }
          event Panel Close {
            n392 = event-data() -> ()  [unwired: 1 in, 3 out]
          }
          event "btn_取消": Value Change {
            n393 = event-data() -> ()  [unwired: 1 in, 5 out]
          }
          event "btn_开始测试": Value Change {
            n394 = event-data() -> ()  [unwired: 1 in, 5 out]
            n395 = stacked-sequence {
              tunnel: w439 -> [_ _ _ w518]
              frame #0 {
                w440 = 0 ("第几组数据")
                n396 = local read "Analog_IN"() -> (w447:string[][])
                n397 = Delete From Array(array=w447, length=1 ("长度"), index (col)=0 ("禁用的索引 (列)")) -> (array with subset deleted=w443:string[][])  [unwired: 1 in, 1 out]
                n398 = for {
                  N: 32 -> [_]
                  tunnel: w443 -> [w450] mode=indexing
                  tunnel: [w449] -> w446 mode=indexing
                  n399 = for {
                    N: 5 -> [_]
                    tunnel: w450 -> [w452] mode=indexing
                    tunnel: [w451] -> w449 mode=indexing
                    n400 = Fract/Exp String To Number(string=w452) -> (number=w451:dbl)  [unwired: 3 in, 1 out]
                  }
                }
                n401 = local write "第几组数据"(w440) -> ()
                n402 = local write "第几个数据"(w440) -> ()
                n403 = local write "同步_1"(0 ("同步_2")) -> ()
                n404 = local write "数组_设定值"(w446) -> ()
              }
              frame #1 {
                n405 = local read "Analog_back"() -> (w455:string[][])
                n406 = local read "Analog_WC"() -> (w454:string[][])
                n407 = for {
                  tunnel: w454 -> [w491] mode=indexing
                  i -> [w490]
                  n408 = for {
                    tunnel: w491 -> [_] mode=indexing
                    tunnel: w490 -> [w495]
                    i -> [w494]
                    n409 = local read "Analog_WC"() -> (w496:string[][])
                    n410 = Replace Array Subset(array=w496, new element="", index (row)=w495, index (col)=w494) -> (w492:string[][])
                    n411 = local write "Analog_WC"(w492) -> ()
                  }
                }
                n412 = for {
                  tunnel: w455 -> [w498] mode=indexing
                  i -> [w497]
                  n413 = for {
                    tunnel: w498 -> [_] mode=indexing
                    tunnel: w497 -> [w502]
                    i -> [w501]
                    n414 = local read "Analog_back"() -> (w503:string[][])
                    n415 = Replace Array Subset(array=w503, new element="", index (row)=w502, index (col)=w501) -> (w499:string[][])
                    n416 = local write "Analog_back"(w499) -> ()
                  }
                }
                n417 = for {
                  N: 32 -> [_]
                  i -> [w457]
                  n418 = case shown="31" w457 {
                    tunnel: cluster{u32, u32}[] [{9868950, 9868950}] -> [w458 w459 w460 w461 w462 w463 w464 w465 w466 w467 w468 w469 w470 w471 w472 w473 w474 w475 w476 w477 w478 w479 w480 w481 w482 w483 w484 w485 w486 w487 w488 w489]
                    frame 0, Default {
                      n419 = property on="light_1" class="Bool (严格)"("Colors [4]"=w458) -> ()  [unwired: 2 in, 2 out]
                    }
                    frame 1 {
                      n420 = property on="light_2" class="Bool (严格)"("Colors [4]"=w459) -> ()  [unwired: 2 in, 2 out]
                    }
                    frame 2 {
                      n421 = property on="light_3" class="Bool (严格)"("Colors [4]"=w460) -> ()  [unwired: 2 in, 2 out]
                    }
                    frame 3 {
                      n422 = property on="light_4" class="Bool (严格)"("Colors [4]"=w461) -> ()  [unwired: 2 in, 2 out]
                    }
                    frame 4 {
                      n423 = property on="light_5" class="Bool (严格)"("Colors [4]"=w462) -> ()  [unwired: 2 in, 2 out]
                    }
                    frame 5 {
                      n424 = property on="light_6" class="Bool (严格)"("Colors [4]"=w463) -> ()  [unwired: 2 in, 2 out]
                    }
                    frame 6 {
                      n425 = property on="light_7" class="Bool (严格)"("Colors [4]"=w464) -> ()  [unwired: 2 in, 2 out]
                    }
                    frame 7 {
                      n426 = property on="light_8" class="Bool (严格)"("Colors [4]"=w465) -> ()  [unwired: 2 in, 2 out]
                    }
                    frame 8 {
                      n427 = property on="light_9" class="Bool (严格)"("Colors [4]"=w466) -> ()  [unwired: 2 in, 2 out]
                    }
                    frame 9 {
                      n428 = property on="light_10" class="Bool (严格)"("Colors [4]"=w467) -> ()  [unwired: 2 in, 2 out]
                    }
                    frame 10 {
                      n429 = property on="light_11" class="Bool (严格)"("Colors [4]"=w468) -> ()  [unwired: 2 in, 2 out]
                    }
                    frame 11 {
                      n430 = property on="light_12" class="Bool (严格)"("Colors [4]"=w469) -> ()  [unwired: 2 in, 2 out]
                    }
                    frame 12 {
                      n431 = property on="light_13" class="Bool (严格)"("Colors [4]"=w470) -> ()  [unwired: 2 in, 2 out]
                    }
                    frame 13 {
                      n432 = property on="light_14" class="Bool (严格)"("Colors [4]"=w471) -> ()  [unwired: 2 in, 2 out]
                    }
                    frame 14 {
                      n433 = property on="light_15" class="Bool (严格)"("Colors [4]"=w472) -> ()  [unwired: 2 in, 2 out]
                    }
                    frame 15 {
                      n434 = property on="light_16" class="Bool (严格)"("Colors [4]"=w473) -> ()  [unwired: 2 in, 2 out]
                    }
                    frame 16 {
                      n435 = property on="light_17" class="Bool (严格)"("Colors [4]"=w474) -> ()  [unwired: 2 in, 2 out]
                    }
                    frame 17 {
                      n436 = property on="light_18" class="Bool (严格)"("Colors [4]"=w475) -> ()  [unwired: 2 in, 2 out]
                    }
                    frame 18 {
                      n437 = property on="light_19" class="Bool (严格)"("Colors [4]"=w476) -> ()  [unwired: 2 in, 2 out]
                    }
                    frame 19 {
                      n438 = property on="light_20" class="Bool (严格)"("Colors [4]"=w477) -> ()  [unwired: 2 in, 2 out]
                    }
                    frame 20 {
                      n439 = property on="light_21" class="Bool (严格)"("Colors [4]"=w478) -> ()  [unwired: 2 in, 2 out]
                    }
                    frame 21 {
                      n440 = property on="light_22" class="Bool (严格)"("Colors [4]"=w479) -> ()  [unwired: 2 in, 2 out]
                    }
                    frame 22 {
                      n441 = property on="light_23" class="Bool (严格)"("Colors [4]"=w480) -> ()  [unwired: 2 in, 2 out]
                    }
                    frame 23 {
                      n442 = property on="light_24" class="Bool (严格)"("Colors [4]"=w481) -> ()  [unwired: 2 in, 2 out]
                    }
                    frame 24 {
                      n443 = property on="light_25" class="Bool (严格)"("Colors [4]"=w482) -> ()  [unwired: 2 in, 2 out]
                    }
                    frame 25 {
                      n444 = property on="light_26" class="Bool (严格)"("Colors [4]"=w483) -> ()  [unwired: 2 in, 2 out]
                    }
                    frame 26 {
                      n445 = property on="light_27" class="Bool (严格)"("Colors [4]"=w484) -> ()  [unwired: 2 in, 2 out]
                    }
                    frame 27 {
                      n446 = property on="light_28" class="Bool (严格)"("Colors [4]"=w485) -> ()  [unwired: 2 in, 2 out]
                    }
                    frame 28 {
                      n447 = property on="light_29" class="Bool (严格)"("Colors [4]"=w486) -> ()  [unwired: 2 in, 2 out]
                    }
                    frame 29 {
                      n448 = property on="light_30" class="Bool (严格)"("Colors [4]"=w487) -> ()  [unwired: 2 in, 2 out]
                    }
                    frame 30 {
                      n449 = property on="light_31" class="Bool (严格)"("Colors [4]"=w488) -> ()  [unwired: 2 in, 2 out]
                    }
                    frame 31 {
                      n450 = property on="light_32" class="Bool (严格)"("Colors [4]"=w489) -> ()  [unwired: 2 in, 2 out]
                    }
                  }
                }
              }
              frame #2 {
                n451 = for {
                  N: 32 -> [_]
                  i -> [w506]
                  n452 = disable-structure shown="禁用" {
                    frame Disabled {
                      n453 = Wait Until Next ms Multiple(millisecond multiple=u32 10 ("毫秒倍数")) -> ()  [unwired: 1 out]
                    }
                    frame Enabled {
                    }
                  }
                  n454 = for {
                    N: 6 -> [_]
                    tunnel: w506 -> [w514]
                    i -> [w511]
                    n455 = Bundle(w514, w511) -> (w510:cluster{i32, i32})  [unwired: 1 in]
                    n456 = Quotient & Remainder(x=w514, y=2) -> (x-y*floor(x/y)=w512:i32)  [unwired: 1 out]
                    n457 = property on="Analog_WC" class="Tbl (严格)"("Active Cell"=w510) -> (error out=w509:errorcluster)  [unwired: 2 in, 1 out]
                    n458 = Equal To 0?(x=w512) -> (x = 0?=w515:bool)
                    n459 = case shown="假" w515 {
                      tunnel: [u32 16448250 u32 15723488] -> w508
                      frame False {
                      }
                      frame True {
                      }
                    }
                    n460 = property on="Analog_WC" class="Tbl (严格)"(error in=w509, "Cell BG Color"=w508) -> ()  [unwired: 1 in, 2 out]
                  }
                }
              }
              frame #3 {
                n461 = local read "A_10"() -> (w548:bool)
                n462 = local read "A_11"() -> (w547:bool)
                n463 = local read "A_12"() -> (w546:bool)
                n464 = local read "A_13"() -> (w545:bool)
                n465 = local read "A_14"() -> (w544:bool)
                n466 = local read "A_15"() -> (w543:bool)
                n467 = local read "A_16"() -> (w542:bool)
                n468 = local read "A_17"() -> (w541:bool)
                n469 = local read "A_18"() -> (w540:bool)
                n470 = local read "A_19"() -> (w539:bool)
                n471 = local read "A_20"() -> (w538:bool)
                n472 = local read "A_21"() -> (w537:bool)
                n473 = local read "A_22"() -> (w536:bool)
                n474 = local read "A_23"() -> (w535:bool)
                n475 = local read "A_24"() -> (w534:bool)
                n476 = local read "A_25"() -> (w533:bool)
                n477 = local read "A_26"() -> (w532:bool)
                n478 = local read "A_27"() -> (w531:bool)
                n479 = local read "A_28"() -> (w530:bool)
                n480 = local read "A_29"() -> (w529:bool)
                n481 = local read "A_30"() -> (w528:bool)
                n482 = local read "A_31"() -> (w527:bool)
                n483 = local read "A_32"() -> (w526:bool)
                n484 = local read "A_1"() -> (w557:bool)
                n485 = local read "A_2"() -> (w556:bool)
                n486 = local read "A_3"() -> (w555:bool)
                n487 = local read "A_4"() -> (w554:bool)
                n488 = local read "A_5"() -> (w553:bool)
                n489 = local read "A_6"() -> (w552:bool)
                n490 = local read "A_7"() -> (w551:bool)
                n491 = local read "A_8"() -> (w550:bool)
                n492 = local read "A_9"() -> (w549:bool)
                n493 = Build Array(w557, w556, w555, w554, w553, w552, w551, w550, w549, w548, w547, w546, w545, w544, w543, w542, w541, w540, w539, w538, w537, w536, w535, w534, w533, w532, w531, w530, w529, w528, w527, w526) -> (w520:bool[])
                n494 = Or Array Elements(Boolean array=w520) -> (logical OR=w525:bool)
                n495 = case shown="真" w525 {
                  tunnel: w518 -> [_ w558]
                  frame False {
                    n496 = call "显示对话框信息"() -> ()  [unwired: 10 in, 2 out]
                  }
                  frame True {
                    n497 = Send Notification(notification="DSP" ("通知"), notifier=w558) -> ()  [unwired: 1 in, 2 out]
                  }
                }
                n498 = local write "数组_选择"(w520) -> ()
                n499 = Initialize Array(FALSE, 32 ("维数大小"), 5 ("维数大小")) -> (w521:bool[][])
                n500 = property on="btn_取消" class="Bool"("DisabledEnum"=T1."Disabled and Grayed Out" ("禁用")) -> ()  [unwired: 2 in, 2 out]
                n501 = local write "合格？"(w521) -> ()
              }
            }
          }
          event "btn_全选": Value Change {
            w560 = TRUE ("单选_AD_1")
            n502 = event-data() -> ()  [unwired: 1 in, 5 out]
            n503 = local write "A_1"(w560) -> ()
            n504 = local write "A_2"(w560) -> ()
            n505 = local write "A_3"(w560) -> ()
            n506 = local write "A_4"(w560) -> ()
            n507 = local write "A_5"(w560) -> ()
            n508 = local write "A_6"(w560) -> ()
            n509 = local write "A_7"(w560) -> ()
            n510 = local write "A_8"(w560) -> ()
            n511 = local write "A_9"(w560) -> ()
            n512 = local write "A_10"(w560) -> ()
            n513 = local write "A_11"(w560) -> ()
            n514 = local write "A_12"(w560) -> ()
            n515 = local write "A_13"(w560) -> ()
            n516 = local write "A_14"(w560) -> ()
            n517 = local write "A_15"(w560) -> ()
            n518 = local write "A_16"(w560) -> ()
            n519 = local write "A_17"(w560) -> ()
            n520 = local write "A_18"(w560) -> ()
            n521 = local write "A_19"(w560) -> ()
            n522 = local write "A_20"(w560) -> ()
            n523 = local write "A_21"(w560) -> ()
            n524 = local write "A_22"(w560) -> ()
            n525 = local write "A_23"(w560) -> ()
            n526 = local write "A_24"(w560) -> ()
            n527 = local write "A_25"(w560) -> ()
            n528 = local write "A_26"(w560) -> ()
            n529 = local write "A_27"(w560) -> ()
            n530 = local write "A_28"(w560) -> ()
            n531 = local write "A_29"(w560) -> ()
            n532 = local write "A_30"(w560) -> ()
            n533 = local write "A_31"(w560) -> ()
            n534 = local write "A_32"(w560) -> ()
          }
          event "btn_反选": Value Change {
            n535 = event-data() -> ()  [unwired: 1 in, 5 out]
            n536 = local read "A_17"() -> (w592:bool)
            n537 = local read "A_18"() -> (w590:bool)
            n538 = local read "A_19"() -> (w588:bool)
            n539 = local read "A_20"() -> (w586:bool)
            n540 = local read "A_21"() -> (w584:bool)
            n541 = local read "A_22"() -> (w582:bool)
            n542 = local read "A_23"() -> (w580:bool)
            n543 = local read "A_24"() -> (w578:bool)
            n544 = local read "A_25"() -> (w576:bool)
            n545 = local read "A_26"() -> (w574:bool)
            n546 = local read "A_27"() -> (w572:bool)
            n547 = local read "A_28"() -> (w570:bool)
            n548 = local read "A_29"() -> (w568:bool)
            n549 = local read "A_30"() -> (w566:bool)
            n550 = local read "A_31"() -> (w564:bool)
            n551 = local read "A_32"() -> (w562:bool)
            n552 = local read "A_1"() -> (w624:bool)
            n553 = local read "A_2"() -> (w622:bool)
            n554 = local read "A_3"() -> (w621:bool)
            n555 = local read "A_4"() -> (w620:bool)
            n556 = local read "A_5"() -> (w619:bool)
            n557 = local read "A_6"() -> (w618:bool)
            n558 = local read "A_7"() -> (w617:bool)
            n559 = local read "A_8"() -> (w616:bool)
            n560 = local read "A_9"() -> (w615:bool)
            n561 = local read "A_10"() -> (w614:bool)
            n562 = local read "A_11"() -> (w613:bool)
            n563 = local read "A_12"() -> (w612:bool)
            n564 = local read "A_13"() -> (w611:bool)
            n565 = local read "A_14"() -> (w610:bool)
            n566 = local read "A_15"() -> (w609:bool)
            n567 = local read "A_16"() -> (w608:bool)
            n568 = Not(x=w624) -> (.not. x?=w623:bool)
            n569 = Not(x=w622) -> (.not. x?=w593:bool)
            n570 = Not(x=w621) -> (.not. x?=w594:bool)
            n571 = Not(x=w620) -> (.not. x?=w595:bool)
            n572 = Not(x=w619) -> (.not. x?=w596:bool)
            n573 = Not(x=w618) -> (.not. x?=w597:bool)
            n574 = Not(x=w617) -> (.not. x?=w598:bool)
            n575 = Not(x=w616) -> (.not. x?=w599:bool)
            n576 = Not(x=w615) -> (.not. x?=w600:bool)
            n577 = Not(x=w614) -> (.not. x?=w601:bool)
            n578 = Not(x=w613) -> (.not. x?=w602:bool)
            n579 = Not(x=w612) -> (.not. x?=w603:bool)
            n580 = Not(x=w611) -> (.not. x?=w604:bool)
            n581 = Not(x=w610) -> (.not. x?=w605:bool)
            n582 = Not(x=w609) -> (.not. x?=w606:bool)
            n583 = Not(x=w608) -> (.not. x?=w607:bool)
            n584 = Not(x=w592) -> (.not. x?=w591:bool)
            n585 = Not(x=w590) -> (.not. x?=w589:bool)
            n586 = Not(x=w588) -> (.not. x?=w587:bool)
            n587 = Not(x=w586) -> (.not. x?=w585:bool)
            n588 = Not(x=w584) -> (.not. x?=w583:bool)
            n589 = Not(x=w582) -> (.not. x?=w581:bool)
            n590 = Not(x=w580) -> (.not. x?=w579:bool)
            n591 = Not(x=w578) -> (.not. x?=w577:bool)
            n592 = Not(x=w576) -> (.not. x?=w575:bool)
            n593 = Not(x=w574) -> (.not. x?=w573:bool)
            n594 = Not(x=w572) -> (.not. x?=w571:bool)
            n595 = Not(x=w570) -> (.not. x?=w569:bool)
            n596 = Not(x=w568) -> (.not. x?=w567:bool)
            n597 = Not(x=w566) -> (.not. x?=w565:bool)
            n598 = Not(x=w564) -> (.not. x?=w563:bool)
            n599 = Not(x=w562) -> (.not. x?=w561:bool)
            n600 = local write "A_1"(w623) -> ()
            n601 = local write "A_2"(w593) -> ()
            n602 = local write "A_3"(w594) -> ()
            n603 = local write "A_4"(w595) -> ()
            n604 = local write "A_5"(w596) -> ()
            n605 = local write "A_6"(w597) -> ()
            n606 = local write "A_7"(w598) -> ()
            n607 = local write "A_8"(w599) -> ()
            n608 = local write "A_9"(w600) -> ()
            n609 = local write "A_10"(w601) -> ()
            n610 = local write "A_11"(w602) -> ()
            n611 = local write "A_12"(w603) -> ()
            n612 = local write "A_13"(w604) -> ()
            n613 = local write "A_14"(w605) -> ()
            n614 = local write "A_15"(w606) -> ()
            n615 = local write "A_16"(w607) -> ()
            n616 = local write "A_17"(w591) -> ()
            n617 = local write "A_18"(w589) -> ()
            n618 = local write "A_19"(w587) -> ()
            n619 = local write "A_20"(w585) -> ()
            n620 = local write "A_21"(w583) -> ()
            n621 = local write "A_22"(w581) -> ()
            n622 = local write "A_23"(w579) -> ()
            n623 = local write "A_24"(w577) -> ()
            n624 = local write "A_25"(w575) -> ()
            n625 = local write "A_26"(w573) -> ()
            n626 = local write "A_27"(w571) -> ()
            n627 = local write "A_28"(w569) -> ()
            n628 = local write "A_29"(w567) -> ()
            n629 = local write "A_30"(w565) -> ()
            n630 = local write "A_31"(w563) -> ()
            n631 = local write "A_32"(w561) -> ()
          }
        }
        n632 = local write "退出？"(w436) -> ()
      }
      n633 = Obtain Notifier(name (unnamed)=w169, notification data type=w169) -> (notifier out=w171:refnum<notifier>, error out=w170:errorcluster)  [unwired: 2 in, 1 out]
      n634 = Obtain Notifier(name (unnamed)=w159, notification data type=w159) -> (notifier out=w158:refnum<notifier>)  [unwired: 2 in, 2 out]
      n635 = while {
        tunnel: w171 -> [w359]
        tunnel: w170 -> [w358]
        tunnel: [w357] -> w168
        tunnel: [w356] -> w167
        tunnel: w158 -> [w355]
        stop <- w361 stop-if-true
        n636 = Wait Until Next ms Multiple(millisecond multiple=u32 10 ("毫秒倍数")) -> ()  [unwired: 1 out]
        n637 = Wait on Notification(notifier=w359, timeout in ms (-1)=20 ("超时毫秒(-1)"), error in (no error)=w358) -> (notifier out=w357:refnum<notifier>, notification=w365:string, error out=w356:errorcluster)  [unwired: 1 in, 1 out]
        n638 = Equal?(x=w365, y="DSP" ("通知")) -> (x = y?=w362:bool)
        n639 = case shown="真" w362 {
          tunnel: w355 -> [_ w366]
          frame False {
          }
          frame True {
            n640 = stacked-sequence {
              tunnel: w366 -> [w367 _]
              frame #0 {
                n641 = for {
                  N: 16 -> [_]
                  tunnel: w367 -> [w369]
                  i -> [w373]
                  n642 = local read "数组_选择"() -> (w376:bool[])
                  n643 = disable-structure shown="禁用" {
                    frame Disabled {
                      n644 = property on="Analog_IN" class="Tbl (严格)"() -> ("Value"=w378:string[][])  [unwired: 2 in, 2 out]
                      n645 = call "表格至数组.vi"("表格控件"=w378) -> ()  [unwired: 10 in, 1 out]
                    }
                    frame Enabled {
                    }
                  }
                  n646 = local read "数组_设定值"() -> (w377:dbl[][])
                  n647 = Add(x=w373, y=16) -> (x+y=w374:i32)
                  n648 = Index Array(array=w376, index #1=w373, index #2=w374) -> (element #1=w371:bool, element #2=w370:bool)
                  n649 = Or(x=w371, y=w370) -> (x .or. y?=w375:bool)
                  n650 = case shown="真" w375 {
                    tunnel: w373 -> [_ w380]
                    tunnel: w377 -> [_ w382]
                    tunnel: w369 -> [_ w379]
                    frame False {
                    }
                    frame True {
                      n651 = Increment(x=w380) -> (x+1=w383:i32)
                      n652 = To Unsigned Byte Integer(number=w383) -> (unsigned 8bit integer=w384:u8)
                      n653 = call "一组模拟量CAN切换开关.vi"("第几组数据"=w384) -> ()  [unwired: 10 in, 1 out]
                      n654 = case shown="真" TRUE {
                        tunnel: w380 -> [_ w386]
                        tunnel: w382 -> [_ w387]
                        tunnel: w379 -> [_ w385]
                        frame False {
                        }
                        frame True {
                          n655 = local write "第几组数据"(w386) -> ()
                          n656 = for {
                            N: 5 -> [_]
                            tunnel: w386 -> [w392]
                            tunnel: w387 -> [w391]
                            tunnel: w385 -> [w389]
                            i -> [w390]
                            n657 = while {
                              tunnel: w392 -> [w401]
                              tunnel: w391 -> [w400]
                              tunnel: w390 -> [w399]
                              tunnel: w389 -> [w393]
                              stop <- w396 stop-if-true
                              n658 = local read "同步_1"() -> (w397:i32)
                              n659 = Wait Until Next ms Multiple(millisecond multiple=u32 10 ("毫秒倍数")) -> ()  [unwired: 1 out]
                              n660 = Equal?(x=w397, y=0) -> (x = y?=w398:bool)
                              n661 = case shown="真" w398 {
                                tunnel: w401 -> [_ w407]
                                tunnel: w400 -> [_ w406]
                                tunnel: w399 -> [_ w405]
                                tunnel: [FALSE w404] -> w396
                                tunnel: w393 -> [_ w403]
                                frame False {
                                }
                                frame True {
                                n662 = stacked-sequence {
                                tunnel: w407 -> [_ w413 _ _ w430 _]
                                tunnel: w406 -> [_ w416 _ _ _ _]
                                tunnel: w405 -> [_ w409 _ _ _ _]
                                tunnel: [_ _ _ _ _ w431] -> w404
                                tunnel: w403 -> [_ _ w419 _ _ _]
                                frame #0 {
                                n663 = Wait (ms)(milliseconds to wait=u32 100) -> ()  [unwired: 1 out]
                                }
                                frame #1 {
                                # "PCI板卡下发模拟量数据"
                                n664 = To Long Integer(number=w413) -> (32bit integer=w412:i32)
                                n665 = local write "第几个数据"(w409) -> ()
                                n666 = Add(x=w412, y=16) -> (x+y=w414:i32)
                                n667 = Index Array(array=w416, index (row) #1=w412, index (col) #1=w409, index (row) #2=w414, index (col) #2=w409) -> (element #1=w411:dbl, element #2=w410:dbl)
                                n668 = Build Array(w411, w410) -> (w417:dbl[])
                                n669 = call "Convert to Dynamic Data"("Array"=w417) -> ("Dynamic Data Type"=w418:dynamicdata)  [unwired: 3 out]
                                n670 = call "DAQNavi Assistant"("data in(DDT)"=w418) -> ()  [unwired: 2 in, 17 out]
                                }
                                frame #2 {
                                n671 = local write "同步_1"(1 ("同步_1")) -> ()
                                n672 = Send Notification(notification="NumCheck" ("通知"), notifier=w419) -> ()  [unwired: 1 in, 2 out]
                                }
                                frame #3 {
                                n673 = Wait (ms)(milliseconds to wait=u32 150) -> ()  [unwired: 1 out]
                                }
                                frame #4 {
                                # "待定"
                                # "待定"
                                # "待定"
                                # "以太网发送读取参数命令"
                                n674 = To Unsigned Word Integer(number=w430) -> (unsigned 16bit integer=w426:u16)
                                n675 = Add(x=w426, y=u16 16) -> (x+y=w427:u16)
                                n676 = Build Array(w426, w427) -> (w429:u16[])
                                n677 = call "UDP发送.vi"("发送数据"=w429, "数据区字长"=u16 2, "报文类型"=u16 2056, "发送方标识"=u16 5397) -> ()  [unwired: 6 in, 1 out]
                                }
                                frame #5 {
                                n678 = local read "同步_1"() -> (w433:i32)
                                n679 = Equal?(x=w433, y=1) -> (x = y?=w431:bool)
                                }
                                }
                                }
                              }
                            }
                          }
                        }
                      }
                    }
                  }
                }
              }
              frame #1 {
                n680 = property on="btn_取消" class="Bool"("DisabledEnum"=T1."Enabled" ("禁用")) -> ()  [unwired: 2 in, 2 out]
              }
            }
          }
        }
        n681 = local read "退出？"() -> (w361:bool)
      }
      n682 = Release Notifier(notifier=w168, error in (no error)=w167) -> ()  [unwired: 1 in, 3 out]
      n683 = Obtain Notifier(name (unnamed)=w166, notification data type=w166) -> (notifier out=w165:refnum<notifier>, error out=w164:errorcluster)  [unwired: 2 in, 1 out]
      n684 = while {
        tunnel: w165 -> [w176]
        tunnel: w164 -> [w175]
        tunnel: [w174] -> w163
        tunnel: [w173] -> w162
        stop <- w172 stop-if-true
        n685 = Wait Until Next ms Multiple(millisecond multiple=u32 10 ("毫秒倍数")) -> ()  [unwired: 1 out]
        n686 = Wait on Notification(notifier=w176, timeout in ms (-1)=20 ("超时毫秒(-1)"), error in (no error)=w175) -> (notifier out=w174:refnum<notifier>, notification=w179:string, error out=w173:errorcluster)  [unwired: 1 in, 1 out]
        n687 = Equal?(x=w179, y="NumCheck" ("通知")) -> (x = y?=w177:bool)
        n688 = case shown="真" w177 {
          frame False {
          }
          frame True {
            w184 = u16 4
            w193 = u16 5397
            # "以太网返回查询到的参数"
            n689 = Build Array(w193, u16 2056, w184) -> (w190:u16[])
            n690 = Build Array(w193, u16 34952, u16 0 ("元素")) -> (w189:u16[])
            n691 = Add(x=w184, y=u16 4) -> (x+y=w182:u16)
            n692 = call "UDP接收.vi"("匹配帧信息_异常"=w189, "长度"=w182, "匹配帧信息_正常"=w190) -> ("异常_找到?"=w186:bool, "接收超时?"=w185:bool, "接收的一帧数据"=w187:u16[], "正常_找到?"=w188:bool)  [unwired: 5 in]
            n693 = case shown="真" w185 {
              frame False {
              }
              frame True {
                n694 = disable-structure shown="禁用" {
                  frame Disabled {
                    n695 = call "超时"() -> ()  [unwired: 10 in, 2 out]
                  }
                  frame Enabled {
                  }
                }
                n696 = local write "同步_1"(0 ("同步_1")) -> ()
              }
            }
            n697 = case shown="真" w188 {
              tunnel: w187 -> [_ w203]
              frame False {
              }
              frame True {
                n698 = stacked-sequence {
                  tunnel: w203 -> [w243 _ _ _]
                  frame #0 {
                    n699 = local read "第几组数据"() -> (w211:i32)
                    n700 = local read "第几个数据"() -> (w206:i32)
                    n701 = local read "数组_设定值"() -> (w237:dbl[][])
                    n702 = local read "数组_选择"() -> (w215:bool[])
                    n703 = Index Array(array=w243, index #1=3 ("索引"), index #2=4 ("索引"), index #3=5 ("索引"), index #4=6 ("索引")) -> (element #1=w222:u16, element #2=w221:u16, element #3=w220:u16, element #4=w219:u16)
                    n704 = local read "第几组数据"() -> (w218:i32)
                    n705 = Add(x=w211, y=16) -> (x+y=w224:i32)
                    n706 = call "U16转换为float.vi"("第几组数据"=w218, "选择?"=w215, "低16位_2"=w219, "高16位_2"=w220, "低16位_1"=w221, "高16位_1"=w222) -> ("反馈值2"=w213:dbl, "反馈值1"=w204:dbl, "反馈值字符_2"=w216:string, "反馈值字符_1"=w217:string)  [unwired: 2 in]
                    n707 = Index Array(array=w237, index (row) #1=w211, index (col) #1=w206, index (row) #2=w224, index (col) #2=w206) -> (element #1=w205:dbl, element #2=w212:dbl)
                    n708 = local read "Analog_back"() -> (w229:string[][])
                    n709 = local read "第几个数据"() -> (w223:i32)
                    n710 = local read "数组_选择"() -> (w214:bool[])
                    n711 = Add(x=w218, y=16) -> (x+y=w227:i32)
                    n712 = call "一个反馈计算误差.vi"("第几组"=w211, "选择?"=w214, "设定值_2"=w212, "设定值_1"=w205, "反馈值_2"=w213, "反馈值_1"=w204) -> ("字符串_误差_2"=w208:string, "字符串_误差_1"=w209:string, "合格_2?"=w207:bool, "合格_1?"=w210:bool)  [unwired: 2 out]
                    n713 = Replace Array Subset(array=w229, new element #1=w217, index (row) #1=w218, index (col) #1=w223, new element #2=w216, index (row) #2=w227, index (col) #2=w223) -> (w228:string[][])
                    n714 = local write "Analog_back"(w228) -> ()
                    n715 = local read "第几个数据"() -> (w225:i32)
                    n716 = local read "Analog_WC"() -> (w234:string[][])
                    n717 = local read "第几组数据"() -> (w232:i32)
                    n718 = Add(x=w232, y=16) -> (x+y=w226:i32)
                    n719 = Replace Array Subset(array=w234, new element #1=w209, index (row) #1=w232, index (col) #1=w225, new element #2=w208, index (row) #2=w226, index (col) #2=w225) -> (w233:string[][])
                    n720 = local read "合格？"() -> (w230:bool[][])
                    n721 = local write "Analog_WC"(w233) -> ()
                    n722 = Replace Array Subset(array=w230, new element #1=w210, index (row) #1=w232, index (col) #1=w225, new element #2=w207, index (row) #2=w226, index (col) #2=w225) -> (w231:bool[][])
                    n723 = local write "合格？"(w231) -> ()
                  }
                  frame #1 {
                    n724 = local read "合格？"() -> (w253:bool[][])
                    n725 = local read "第几组数据"() -> (w247:i32)
                    n726 = Add(x=w247, y=16) -> (x+y=w246:i32)
                    n727 = Index Array(array=w253, index (row) #1=w247, index (row) #2=w246) -> (element #1=w256:bool[], element #2=w250:bool[])  [unwired: 2 in]
                    n728 = And Array Elements(Boolean array=w256) -> (logical AND=w251:bool)
                    n729 = And Array Elements(Boolean array=w250) -> (logical AND=w249:bool)
                    n730 = local read "数组_选择"() -> (w248:bool[])
                    n731 = Index Array(array=w248, index #1=w247, index #2=w246) -> (element #1=w245:bool, element #2=w244:bool)
                    n732 = case shown="真" w245 {
                      tunnel: [cluster{u32, u32}[] [{12369084, 12369084}] w264] -> w255
                      tunnel: w251 -> [_ w263]
                      frame False {
                      }
                      frame True {
                        n733 = case shown="真" w263 {
                          tunnel: [cluster{u32, u32}[] [{16730410, 16711680}] cluster{u32, u32}[] [{61205, 6618880}]] -> w264
                          frame False {
                          }
                          frame True {
                          }
                        }
                      }
                    }
                    n734 = case shown="真" w244 {
                      tunnel: [cluster{u32, u32}[] [{12369084, 12369084}] w259] -> w252
                      tunnel: w249 -> [_ w258]
                      frame False {
                      }
                      frame True {
                        n735 = case shown="真" w258 {
                          tunnel: [cluster{u32, u32}[] [{16730410, 16711680}] cluster{u32, u32}[] [{61205, 6618880}]] -> w259
                          frame False {
                          }
                          frame True {
                          }
                        }
                      }
                    }
                    n736 = case shown="31" w247 {
                      tunnel: w255 -> [w299 w300 w301 w302 w303 w304 w305 w306 w307 w308 w309 w310 w311 w312 w313 w314 w315 w316 w317 w318 w319 w320 w321 w322 w323 w324 w325 w326 w327 w328 w329 w330]
                      frame 0, Default {
                        n737 = property on="light_1" class="Bool (严格)"("Colors [4]"=w299) -> ()  [unwired: 2 in, 2 out]
                      }
                      frame 1 {
                        n738 = property on="light_2" class="Bool (严格)"("Colors [4]"=w300) -> ()  [unwired: 2 in, 2 out]
                      }
                      frame 2 {
                        n739 = property on="light_3" class="Bool (严格)"("Colors [4]"=w301) -> ()  [unwired: 2 in, 2 out]
                      }
                      frame 3 {
                        n740 = property on="light_4" class="Bool (严格)"("Colors [4]"=w302) -> ()  [unwired: 2 in, 2 out]
                      }
                      frame 4 {
                        n741 = property on="light_5" class="Bool (严格)"("Colors [4]"=w303) -> ()  [unwired: 2 in, 2 out]
                      }
                      frame 5 {
                        n742 = property on="light_6" class="Bool (严格)"("Colors [4]"=w304) -> ()  [unwired: 2 in, 2 out]
                      }
                      frame 6 {
                        n743 = property on="light_7" class="Bool (严格)"("Colors [4]"=w305) -> ()  [unwired: 2 in, 2 out]
                      }
                      frame 7 {
                        n744 = property on="light_8" class="Bool (严格)"("Colors [4]"=w306) -> ()  [unwired: 2 in, 2 out]
                      }
                      frame 8 {
                        n745 = property on="light_9" class="Bool (严格)"("Colors [4]"=w307) -> ()  [unwired: 2 in, 2 out]
                      }
                      frame 9 {
                        n746 = property on="light_10" class="Bool (严格)"("Colors [4]"=w308) -> ()  [unwired: 2 in, 2 out]
                      }
                      frame 10 {
                        n747 = property on="light_11" class="Bool (严格)"("Colors [4]"=w309) -> ()  [unwired: 2 in, 2 out]
                      }
                      frame 11 {
                        n748 = property on="light_12" class="Bool (严格)"("Colors [4]"=w310) -> ()  [unwired: 2 in, 2 out]
                      }
                      frame 12 {
                        n749 = property on="light_13" class="Bool (严格)"("Colors [4]"=w311) -> ()  [unwired: 2 in, 2 out]
                      }
                      frame 13 {
                        n750 = property on="light_14" class="Bool (严格)"("Colors [4]"=w312) -> ()  [unwired: 2 in, 2 out]
                      }
                      frame 14 {
                        n751 = property on="light_15" class="Bool (严格)"("Colors [4]"=w313) -> ()  [unwired: 2 in, 2 out]
                      }
                      frame 15 {
                        n752 = property on="light_16" class="Bool (严格)"("Colors [4]"=w314) -> ()  [unwired: 2 in, 2 out]
                      }
                      frame 16 {
                        n753 = property on="light_17" class="Bool (严格)"("Colors [4]"=w315) -> ()  [unwired: 2 in, 2 out]
                      }
                      frame 17 {
                        n754 = property on="light_18" class="Bool (严格)"("Colors [4]"=w316) -> ()  [unwired: 2 in, 2 out]
                      }
                      frame 18 {
                        n755 = property on="light_19" class="Bool (严格)"("Colors [4]"=w317) -> ()  [unwired: 2 in, 2 out]
                      }
                      frame 19 {
                        n756 = property on="light_20" class="Bool (严格)"("Colors [4]"=w318) -> ()  [unwired: 2 in, 2 out]
                      }
                      frame 20 {
                        n757 = property on="light_21" class="Bool (严格)"("Colors [4]"=w319) -> ()  [unwired: 2 in, 2 out]
                      }
                      frame 21 {
                        n758 = property on="light_22" class="Bool (严格)"("Colors [4]"=w320) -> ()  [unwired: 2 in, 2 out]
                      }
                      frame 22 {
                        n759 = property on="light_23" class="Bool (严格)"("Colors [4]"=w321) -> ()  [unwired: 2 in, 2 out]
                      }
                      frame 23 {
                        n760 = property on="light_24" class="Bool (严格)"("Colors [4]"=w322) -> ()  [unwired: 2 in, 2 out]
                      }
                      frame 24 {
                        n761 = property on="light_25" class="Bool (严格)"("Colors [4]"=w323) -> ()  [unwired: 2 in, 2 out]
                      }
                      frame 25 {
                        n762 = property on="light_26" class="Bool (严格)"("Colors [4]"=w324) -> ()  [unwired: 2 in, 2 out]
                      }
                      frame 26 {
                        n763 = property on="light_27" class="Bool (严格)"("Colors [4]"=w325) -> ()  [unwired: 2 in, 2 out]
                      }
                      frame 27 {
                        n764 = property on="light_28" class="Bool (严格)"("Colors [4]"=w326) -> ()  [unwired: 2 in, 2 out]
                      }
                      frame 28 {
                        n765 = property on="light_29" class="Bool (严格)"("Colors [4]"=w327) -> ()  [unwired: 2 in, 2 out]
                      }
                      frame 29 {
                        n766 = property on="light_30" class="Bool (严格)"("Colors [4]"=w328) -> ()  [unwired: 2 in, 2 out]
                      }
                      frame 30 {
                        n767 = property on="light_31" class="Bool (严格)"("Colors [4]"=w329) -> ()  [unwired: 2 in, 2 out]
                      }
                      frame 31 {
                        n768 = property on="light_32" class="Bool (严格)"("Colors [4]"=w330) -> ()  [unwired: 2 in, 2 out]
                      }
                    }
                    n769 = case shown="31" w246 {
                      tunnel: w252 -> [w267 w268 w269 w270 w271 w272 w273 w274 w275 w276 w277 w278 w279 w280 w281 w282 w283 w284 w285 w286 w287 w288 w289 w290 w291 w292 w293 w294 w295 w296 w297 w298]
                      frame 0, Default {
                        n770 = property on="light_1" class="Bool (严格)"("Colors [4]"=w267) -> ()  [unwired: 2 in, 2 out]
                      }
                      frame 1 {
                        n771 = property on="light_2" class="Bool (严格)"("Colors [4]"=w268) -> ()  [unwired: 2 in, 2 out]
                      }
                      frame 2 {
                        n772 = property on="light_3" class="Bool (严格)"("Colors [4]"=w269) -> ()  [unwired: 2 in, 2 out]
                      }
                      frame 3 {
                        n773 = property on="light_4" class="Bool (严格)"("Colors [4]"=w270) -> ()  [unwired: 2 in, 2 out]
                      }
                      frame 4 {
                        n774 = property on="light_5" class="Bool (严格)"("Colors [4]"=w271) -> ()  [unwired: 2 in, 2 out]
                      }
                      frame 5 {
                        n775 = property on="light_6" class="Bool (严格)"("Colors [4]"=w272) -> ()  [unwired: 2 in, 2 out]
                      }
                      frame 6 {
                        n776 = property on="light_7" class="Bool (严格)"("Colors [4]"=w273) -> ()  [unwired: 2 in, 2 out]
                      }
                      frame 7 {
                        n777 = property on="light_8" class="Bool (严格)"("Colors [4]"=w274) -> ()  [unwired: 2 in, 2 out]
                      }
                      frame 8 {
                        n778 = property on="light_9" class="Bool (严格)"("Colors [4]"=w275) -> ()  [unwired: 2 in, 2 out]
                      }
                      frame 9 {
                        n779 = property on="light_10" class="Bool (严格)"("Colors [4]"=w276) -> ()  [unwired: 2 in, 2 out]
                      }
                      frame 10 {
                        n780 = property on="light_11" class="Bool (严格)"("Colors [4]"=w277) -> ()  [unwired: 2 in, 2 out]
                      }
                      frame 11 {
                        n781 = property on="light_12" class="Bool (严格)"("Colors [4]"=w278) -> ()  [unwired: 2 in, 2 out]
                      }
                      frame 12 {
                        n782 = property on="light_13" class="Bool (严格)"("Colors [4]"=w279) -> ()  [unwired: 2 in, 2 out]
                      }
                      frame 13 {
                        n783 = property on="light_14" class="Bool (严格)"("Colors [4]"=w280) -> ()  [unwired: 2 in, 2 out]
                      }
                      frame 14 {
                        n784 = property on="light_15" class="Bool (严格)"("Colors [4]"=w281) -> ()  [unwired: 2 in, 2 out]
                      }
                      frame 15 {
                        n785 = property on="light_16" class="Bool (严格)"("Colors [4]"=w282) -> ()  [unwired: 2 in, 2 out]
                      }
                      frame 16 {
                        n786 = property on="light_17" class="Bool (严格)"("Colors [4]"=w283) -> ()  [unwired: 2 in, 2 out]
                      }
                      frame 17 {
                        n787 = property on="light_18" class="Bool (严格)"("Colors [4]"=w284) -> ()  [unwired: 2 in, 2 out]
                      }
                      frame 18 {
                        n788 = property on="light_19" class="Bool (严格)"("Colors [4]"=w285) -> ()  [unwired: 2 in, 2 out]
                      }
                      frame 19 {
                        n789 = property on="light_20" class="Bool (严格)"("Colors [4]"=w286) -> ()  [unwired: 2 in, 2 out]
                      }
                      frame 20 {
                        n790 = property on="light_21" class="Bool (严格)"("Colors [4]"=w287) -> ()  [unwired: 2 in, 2 out]
                      }
                      frame 21 {
                        n791 = property on="light_22" class="Bool (严格)"("Colors [4]"=w288) -> ()  [unwired: 2 in, 2 out]
                      }
                      frame 22 {
                        n792 = property on="light_23" class="Bool (严格)"("Colors [4]"=w289) -> ()  [unwired: 2 in, 2 out]
                      }
                      frame 23 {
                        n793 = property on="light_24" class="Bool (严格)"("Colors [4]"=w290) -> ()  [unwired: 2 in, 2 out]
                      }
                      frame 24 {
                        n794 = property on="light_25" class="Bool (严格)"("Colors [4]"=w291) -> ()  [unwired: 2 in, 2 out]
                      }
                      frame 25 {
                        n795 = property on="light_26" class="Bool (严格)"("Colors [4]"=w292) -> ()  [unwired: 2 in, 2 out]
                      }
                      frame 26 {
                        n796 = property on="light_27" class="Bool (严格)"("Colors [4]"=w293) -> ()  [unwired: 2 in, 2 out]
                      }
                      frame 27 {
                        n797 = property on="light_28" class="Bool (严格)"("Colors [4]"=w294) -> ()  [unwired: 2 in, 2 out]
                      }
                      frame 28 {
                        n798 = property on="light_29" class="Bool (严格)"("Colors [4]"=w295) -> ()  [unwired: 2 in, 2 out]
                      }
                      frame 29 {
                        n799 = property on="light_30" class="Bool (严格)"("Colors [4]"=w296) -> ()  [unwired: 2 in, 2 out]
                      }
                      frame 30 {
                        n800 = property on="light_31" class="Bool (严格)"("Colors [4]"=w297) -> ()  [unwired: 2 in, 2 out]
                      }
                      frame 31 {
                        n801 = property on="light_32" class="Bool (严格)"("Colors [4]"=w298) -> ()  [unwired: 2 in, 2 out]
                      }
                    }
                  }
                  frame #2 {
                    n802 = local read "第几组数据"() -> (w334:i32)
                    n803 = Add(x=w334, y=16) -> (x+y=w336:i32)
                    n804 = local read "第几个数据"() -> (w338:i32)
                    n805 = local read "合格？"() -> (w339:bool[][])
                    n806 = local read "数组_选择"() -> (w337:bool[])
                    n807 = Index Array(array=w339, index (row) #1=w334, index (col) #1=w338, index (row) #2=w336, index (col) #2=w338) -> (element #1=w335:bool, element #2=w331:bool)
                    n808 = Index Array(array=w337, index #1=w334, index #2=w336) -> (element #1=w333:bool, element #2=w332:bool)
                    n809 = case shown="真" w333 {
                      tunnel: w338 -> [_ w350]
                      tunnel: w335 -> [_ w349]
                      tunnel: w334 -> [_ w348]
                      frame False {
                      }
                      frame True {
                        n810 = call "误差表格颜色.vi"("合格？"=w349, "第几组"=w348) -> ("颜色"=w347:u32)  [unwired: 9 in]
                        n811 = Bundle("第几组数据"=w348, "第几个数据"=w350) -> (w352:cluster{"第几组数据":i32, "第几个数据":i32})  [unwired: 1 in]
                        n812 = property on="Analog_WC" class="Tbl (严格)"("Active Cell"=w352) -> (error out=w351:errorcluster)  [unwired: 2 in, 1 out]
                        n813 = property on="Analog_WC" class="Tbl (严格)"(error in=w351, "Cell BG Color"=w347) -> ()  [unwired: 1 in, 2 out]
                      }
                    }
                    n814 = case shown="真" w332 {
                      tunnel: w338 -> [_ w344]
                      tunnel: w336 -> [_ w343]
                      tunnel: w331 -> [_ w341]
                      frame False {
                      }
                      frame True {
                        n815 = Bundle(w343, "第几个数据"=w344) -> (w345:cluster{i32, "第几个数据":i32})  [unwired: 1 in]
                        n816 = call "误差表格颜色.vi"("合格？"=w341, "第几组"=w343) -> ("颜色"=w342:u32)  [unwired: 9 in]
                        n817 = property on="Analog_WC" class="Tbl (严格)"("Active Cell"=w345) -> (error out=w346:errorcluster)  [unwired: 2 in, 1 out]
                        n818 = property on="Analog_WC" class="Tbl (严格)"(error in=w346, "Cell BG Color"=w342) -> ()  [unwired: 1 in, 2 out]
                      }
                    }
                  }
                  frame #3 {
                    n819 = flat-sequence {
                      frame #0 {
                        n820 = Wait Until Next ms Multiple(millisecond multiple=u32 100) -> ()  [unwired: 1 out]
                      }
                      frame #1 {
                        n821 = local write "同步_1"(0 ("同步_1")) -> ()
                      }
                    }
                  }
                }
              }
            }
            n822 = case shown="真" w186 {
              frame False {
              }
              frame True {
                # "第几个"
                # "第几组"
                n823 = local read "第几个数据"() -> (w197:i32)
                n824 = local read "第几组数据"() -> (w199:i32)
                n825 = Increment(x=w199) -> (x+1=w200:i32)
                n826 = Increment(x=w197) -> (x+1=w198:i32)
                n827 = Format Into String(format string="第%d组%d个数据反馈失败（UDP）" ("Message"), w200, w198) -> (resulting string=w201:string)  [unwired: 2 in, 1 out]
                n828 = call "显示对话框信息2"("Message"=w201) -> ()  [unwired: 9 in, 2 out]
                n829 = local write "同步_1"(0 ("同步_1")) -> ()
              }
            }
          }
        }
        n830 = local read "退出？"() -> (w172:bool)
      }
      n831 = Release Notifier(notifier=w163, error in (no error)=w162) -> ()  [unwired: 1 in, 3 out]
    }
  }
